vi "Power_Correlation9.vi"() -> ()   [LabVIEW 2021]
doc: "This VI opens a datalog file created with Write Datalog File Example.vi, reads one record at a time from the file until all are read, then closes the file and checks for errors. The record is a cluster containing a string and an array of single precision numbers."
uses:
  <vilib>/Analysis/2dsp.llb/Decimate (single shot, DBL).vi
  <vilib>/Analysis/baseanly.llb/Mean (DBL).vi
  Plot Routines.llb/Plot Globals.vi
  Response Analysis.llb/Analysis Globals.vi
  Display_Analysis.llb/Display & Avg Globals.vi
  Power_Correlation Utilities.llb/PowerCorrelation_globals.vi
  <vilib>/Analysis/NI_AALPro.lvlib
  <vilib>/Analysis/NI_AALBase.lvlib
panel:
  out "Trace B units":string
  out "Trace A units":string
  in  "Trace # 2":u8
  in  "Traces\nmV to uV":bool
  in  "redux factor":i32=30
  in  "sample rate redux of graph 2":bool
  out "Strings":T1
  out "Original Traces - all Chan":T2(array[cluster])
  out "Stat Results_Mean":T3
  in  "box filter graph":bool
  in  "single chan":bool=TRUE
  in  "Do Stats":bool
  in  "5 SD mark":bool
  out "Median Stats":T4
  out "Means":dbl[](array[numeric])
  in  "Pair":i32[](array[numeric])=[0, 1]
  in  "Export":bool
  in  "Value":enum16{"avg", "max", "min"}(ring)
  in  "Mode":enum16{"Indiv", "Mean SE"}(ring)
  in  "Analysis Transform":enum16{"None", "Log10"}(ring)
  out "Stat Plot":cluster{dbl[], dbl[]}[](graph)
  in  "Last #":i32=5
  in  "Shift by -500 except last traces":bool
  out "NewVal 2":variant
  out "Dual Parameters":T5 {"Depth B" format="%.2f"; "Depth A" format="%.2f"; "Cap B" format="%.2f"; "Cap A" format="%.2f"; "Comp B" format="%.2f"; "Comp A" format="%.2f"; "Extra Stim Mag B" format="%.2f"; "Extra Stim Mag A" format="%.2f"; "extra amp b" format="%.2f"; "extra amp a" format="%.2f"; "extra offset b" format="%.2f"; "extra offset a/cur" format="%.2f"; "extra dur" format="%.2f"; "extra mode" format="%.2f"; "Intra Stim Mag B" format="%.2f"; "Intra Stim Mag A" format="%.2f"; "Step Delay (sim)" format="%.2f"; "Step Amp B" format="%.2f"; "Rest Pot-B(mV)" format="%.2f"; "Rest Pot-A(mV)" format="%.2f"; "SR-B (MOhm)" format="%.2f"; "SR-A (MOhm)" format="%.2f"; "Clamp Level-B" format="%.2f"; "Clamp Level-A" format="%.2f"; "Gain-B" format="%.2f"; "Step/AI Offset(ms)" format="%.2f"; "Gain-A" format="%.2f"; "Post Stim Dur (ms)" format="%.2f"; "Test Interval(sec)" format="%.2f"; "Step Dur(ms)" format="%.2f"; "Step Amp" format="%.2f"; "Stim/AI Offset(ms)" format="%.2f"; "Pulse Number" format="%.2f"; "Pulse Interval(ms)" format="%.2f"; "Ext Stim Path" format="%.2f"; "Clamp Mode" format="%.2f"; "Current Rec Config" format="%.2f"; "Test Type" format="%.2f"}
  out "Analysis Notes":string
  in  "Trace Processing Params":T6={"X-Unit Factor"=enum."1", "dt change factor"=enum."1", "Box Filter Width"=5, "Filter"=enum."FIR lowpass", "Filter High Cut-off (Hz)"=0.2, "Filter Low Cut-off (Hz)"=300.0} {"Filter Low Cut-off (Hz)" format="%.2f"; "Filter High Cut-off (Hz)" format="%.2f"}
  in  "File Info":T7
  in  "Accumulate Func Plots":bool
  in  "Do Function":bool
  in  "Function":T8(ring)
  in  "cut mode":enum16{"Include", "Exclude"}(ring)
  out "dy B":sgl format="%.3f"
  out "dy A":sgl format="%.3f"
  out "File Paths":T9={"Data Path"=path "C:/", "Anal Path"=path "C:/", "File Path List"=[], "Listfile Path"=path "C:/", "Auto Anal Path"=path "C:/"}
  in  "Display Type":enum16{"Stim&Rec", "Dual", "Multi4", "Mapper"}(ring)=enum."Dual"
  in  "Trace B":T10(ring)=enum."File Tr 1"
  in  "Trace A":T10(ring)
  in  "Load Cursor Wind":bool
  in  "Dump Cursor Wind":bool
  in  "rectify":bool
  in  "Up State Analysis":bool
  in  "Export Name":string
  in  "Function post process":T11={"Freq range"={"min"=0.0, "max"=2000.0}, "Normalization"=enum."None", "Filter"={"Enabled"=FALSE, "Cutoff (cyc/Hz or Hz)"=0.4}} {"Filter"."Cutoff (cyc/Hz or Hz)" min=0 max=1000 step=0.0001 format="%.6f"; "Freq range"."max" format="%.2f"; "Freq range"."min" format="%.2f"}
  in  "Copy cursor window":bool
  in  "Func Mode":enum16{"Trace #", "Trace Ch"}(ring)=enum."Trace Ch"
  in  "Correlation Params":bool
  in  "Shuffle Trace":bool
  in  "cursor func":enum16{"2 filter", "+- 10%", "+- 5%", "+-2"}(ring)
  in  "cursors":bool
  in  "Func Type":enum16{"avg", "sum", "norm"}(ring)
  out "CV B":sgl=0.1 min=0 max=1 format="%.2f"
  out "CV A":sgl=0.1 min=0 max=1 format="%.2f"
  in  "Max Interval":sgl=1000.0 min=0 max=10000 format="%.2f"
  in  "Int Bin":sgl=1.0 min=0 max=100 format="%.2f"
  in  "AP Fract":sgl=0.1 min=0 max=1 format="%.2f"
  in  "AP Mode":enum16{"cor", "coh", "Int/AP"}(ring)
  in  "Zoom":bool
  in  "Cursor Near Spike":bool
  in  "Window":enum16{"all", "cursors"}(ring)
  in  "Spike Times B":T12(array[cluster]) {"t0" format="%.2f"; "Length (ms)" format="%.2f"; "Data" format="%.2f"}
  in  "Init Wind":bool
  in  "Spikes Times A":T12(array[cluster]) {"t0" format="%.2f"; "Length (ms)" format="%.2f"; "Data" format="%.2f"}
  in  "AP Time Course":bool
  in  "Add trace":bool
  in  "AP Freq Mode":enum16{"rates", "dif/avg", "all"}(ring)
  in  "AP Freq vs Time":bool
  in  "^2 four wind":bool
  out "Ran AP Cor":sgl format="%.3f"
  in  "Graph Mode":enum16{"Points", "Max", "Min"}(ring)=enum."Max"
  in  "Coord":enum16{"y", "z"}(ring)=enum."z"
  in  "Cursor Slave\nTime Course":bool
  in  "Graph Data":bool
  in  "Time Course Window":sgl=100.0 format="%.2f"
  in  "Function":T13(ring)
  in  "Init Data":bool
  out "y":sgl[](array[numeric]) format="%.2f"
  out "x":sgl[](array[numeric]) format="%.2f"
  out "Data":sgl[](array[numeric]) format="%.2f"
  in  "Add Datum":bool
  in  "Time Course Focus":enum16{"1", "2"}(ring)
  out "Time Course 2":sgl[][](graph)
  in  "Time Course Increment":i32=25
  in  "Time Course":bool
  out "Time Course 1":sgl[][](graph)
  in  "Spectrum Source":enum16{"Trace", "Function"}(ring)
  out "Function Units = ms?":bool
  in  "Filter":bool
  in  "Trace #":u8
  in  "Operate":bool
  in  "oper2":u8
  in  "oper1":u8
  in  "operation":T14(ring)=enum."mult"
  in  "Match dx read":bool
  out "dF":sgl=1.0 min=0 max=1000 step=0.1 format="%.3f"
  in  "Offset/Sc/Ph":sgl format="%.4f"
  in  "Component Num":i32
  in  "Function":T15(ring)
  out "Fixed Window Size":sgl=2000.0 format="%.2f"
  out "Window Size":sgl format="%.2f"
  in  "Fix Wind Size":bool
  in  "cut traces":bool
  in  "Normalization":enum16{"None", "Variance", "Sample Num"}(ring)=enum."Variance"
  in  "Assign Cursors In Plot":bool
  in  "One Cursor Window":bool=TRUE
  out "Cursor Windows by Trace":cluster{"start":dbl, "end":dbl}[](array[cluster]) {"end" format="%.1f"; "start" format="%.1f"}
  in  "Upper Factor":sgl=1.8 format="%.1f"
  in  "Lower Factor":sgl=1.4 format="%.1f"
  in  "Make window wrt Yel Cursor":bool
  out "Delta X":sgl format="%.2f"
  out "Graph 2 - cursor 0 x":sgl format="%.2f"
  out "Graph 2 - cursor 1 x":sgl format="%.2f"
  out "SD B":sgl format="%.5f"
  out "SD A":sgl format="%.5f"
  in  "scale":bool
  in  "Correllation Func":enum16{"labview", "Jay's"}(ring)=enum."Jay's"
  out "Window Avg":sgl format="%.8f"
  in  "Window Func":bool
  in  "Avg Pts":bool
  out "Delta Y":sgl format="%.3f"
  out "Pts Avg":sgl format="%.2f"
  in  "Get Red Cursonr Pts":bool
  in  "Pts Around Yellow cursor":sgl[](array[numeric]) format="%.1f"
  in  "Offset Traces":bool
  in  "Cutoff (cyc/Hz or Hz)":sgl=0.1 min=0 max=1000 step=0.0001 format="%.6f"
  out "Message":string
  in  "Filter Function":bool
  in  "Export Graph":T16(ring)
  in  "Fourier mode":bool
  in  "expand":bool
  in  "zoom":bool
  in  "Corr Func":enum16{"Auto", "Cross"}(ring)=enum."Cross"
  in  "Window Size (ms)":sgl=400.0 step=1 format="%.2f"
  in  "Set to B X-Axis":bool
  in  "Set to A X-Axis":bool
  in  "Prog Info":bool
  out "x-axis":string
  out "y-axis":string
  out "Window Constants":cluster{"Eq Noise BW":ext, "Coherent Gain":ext} {"Coherent Gain" format="%.2f"; "Eq Noise BW" format="%.2f"}
  in  "window":T17(ring)=enum."Hanning"
  out "samp/sec":sgl format="%.2f"
  in  "1/2 sample rate":bool
  in  "Std Function Parameters":T18={"Function"=2, "Mag/Phase"=0, "Magnitude Unit"=3, "Phase Unit"=0, " Log dB or Linear"=0} {"Log dB or Linear" items=["Linear", "dB", "dBm"]; "Phase Unit" items=["Degrees", "Radians"]; "Magnitude Unit" items=["Vrms", "Vpk", "Vrms^2", "Vpk^2", "Vrms/rtHz", "Vpk/rtHz", "Vrms^2/Hz", "Vpk^2/Hz"]; "Mag/Phase" items=["Magnitude", "Phase"]; "Function" items=["Time Waveform", "Amplitude Spectrum", "Power Spectrum", "Cross Power Spectrum", "Frequency Response", "Coherence", "Impulse Response"]}
  out "Focus Trace B":cluster{"T0":sgl, "Delta T":sgl, "Data":sgl[][]} {"Data" format="%.2f"; "Delta T" format="%.6f"; "T0" format="%.6f"}
  out "Focus Trace A":cluster{"T0":sgl, "Delta T":sgl, "Data":sgl[][]} {"Data" format="%.2f"; "Delta T" format="%.6f"; "T0" format="%.6f"}
  out "Old Focus":i32
  in  "Trace Ch Reference":enum16{"0", "1", "2", "3"}(ring)
  out "Trace B":T19(graph)={"T0"=0.0, "delta T"=0.19999999, "Individual Data Sweeps"=[]}
  in  "Focus":i32
  in  "Focus Mode":bool
  in  "Plot Flags 2":bool[](array[boolean])
  in  "Show All":bool
  in  "Trace Export":bool
  out "Graph 2":cluster{"T0":sgl, "delta T":sgl, sgl[][]}(graph)={"T0"=1.1399999, "delta T"=0.0001, []}
  in  "Load List File":bool
  in  "Get File List":bool
  in  "File Path List":cluster{"FilePath":path, "focus":bool}[](array[cluster])
  in  "Quit":bool
  out "Trace A":T19(graph)={"T0"=0.0, "delta T"=0.19999999, "Individual Data Sweeps"=[]}
  # "function\nInt Hist A\nInt Hist B"
  # "V=mV"
  # "Function Operations"
  # "Focus/Graph"
  # "MW, 1.282 = 0.2, 1.645 = 0.1, 1.960 = .05, 2.326 =.02, 2.576 = .01, 2.807 = .005, 3.090 = .002, 3.291 = .001"
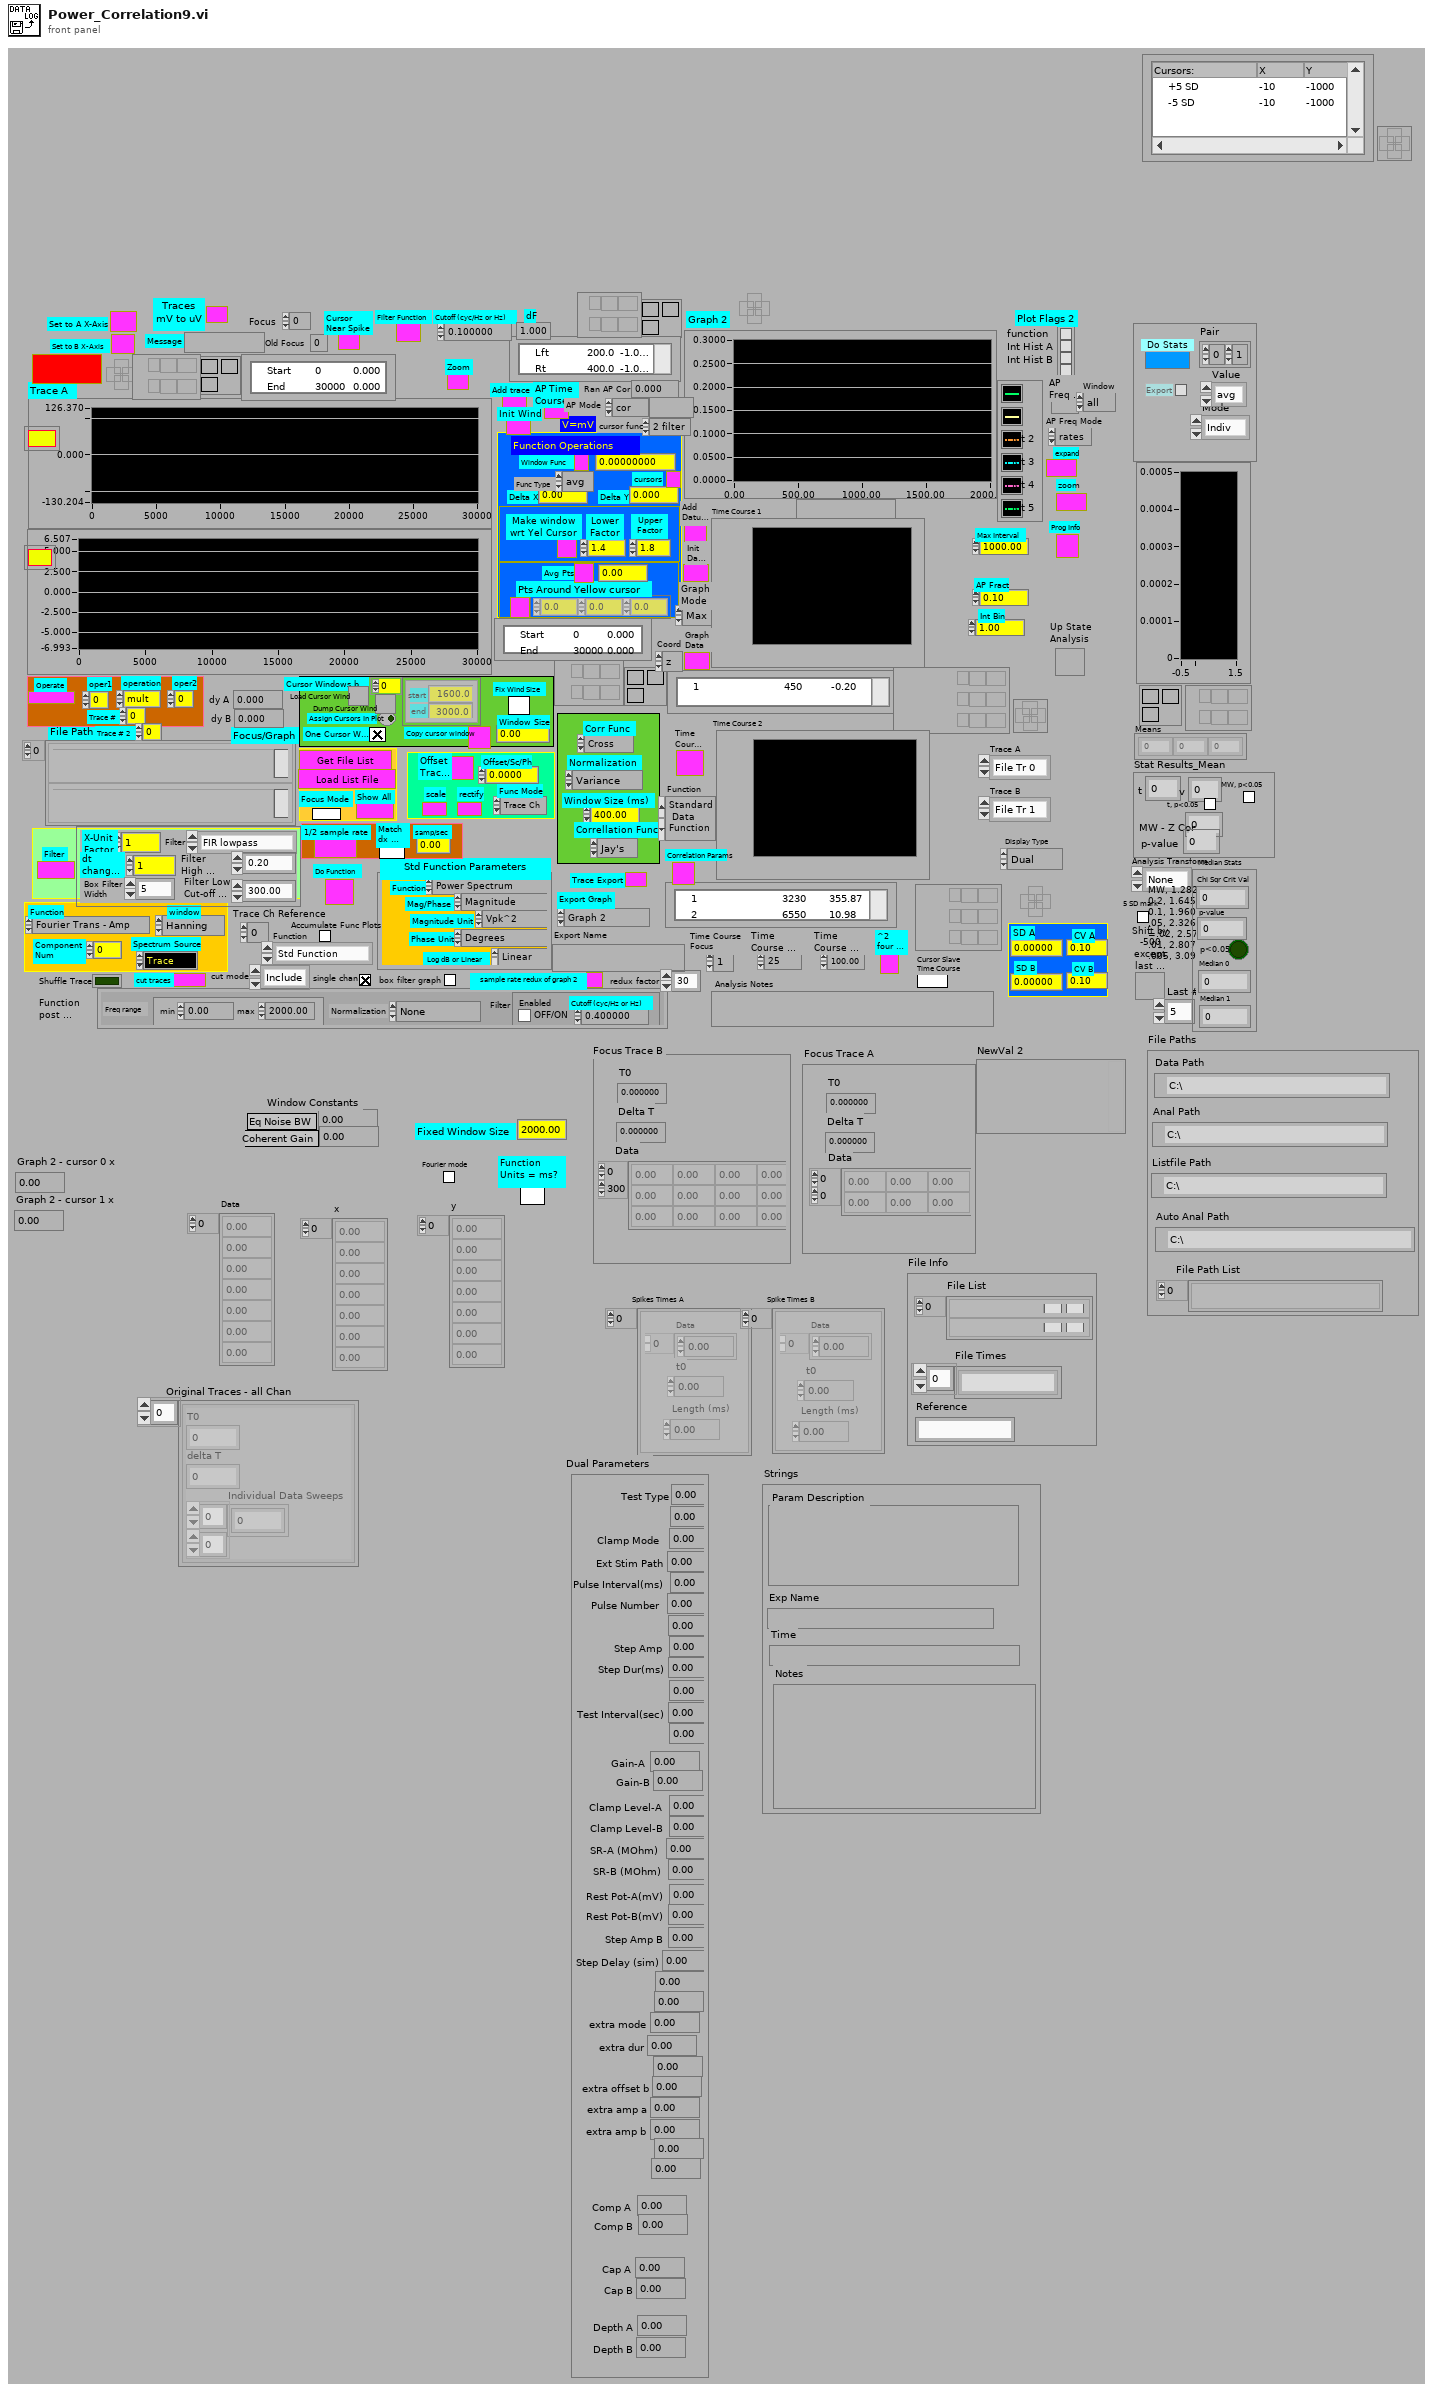
[diagram p1: front panel]
types:
  T1 = cluster{"Param Description":string, "Exp Name":string, "Time":string, "Notes":string}
  T2 = cluster{"T0":sgl, "delta T":sgl, "Individual Data Sweeps":sgl[][]}[]
  T3 = cluster{"t":dbl, "v":i32, "t, p<0.05":bool, "MW - Z Cor":dbl, "MW, p<0.05":bool, "p-value":dbl}
  T4 = cluster{"Chi Sqr Crit Val":dbl, "p-value":dbl, "p<0.05":bool, "Median 0":dbl, "Median 1":dbl}
  T5 = cluster{"Test Type":sgl, "Current Rec Config":sgl, "Clamp Mode":sgl, "Ext Stim Path":sgl, "Pulse Interval(ms)":sgl, "Pulse Number":sgl, "Stim/AI Offset(ms)":sgl, "Step Amp":sgl, "Step Dur(ms)":sgl, "Step/AI Offset(ms)":sgl, "Test Interval(sec)":sgl, "Post Stim Dur (ms)":sgl, "Gain-A":sgl, "Gain-B":sgl, "Clamp Level-A":sgl, "Clamp Level-B":sgl, "SR-A (MOhm)":sgl, "SR-B (MOhm)":sgl, "Rest Pot-A(mV)":sgl, "Rest Pot-B(mV)":sgl, "Step Amp B":sgl, "Step Delay (sim)":sgl, "Intra Stim Mag A":sgl, "Intra Stim Mag B":sgl, "extra mode":sgl, "extra dur":sgl, "extra offset a/cur":sgl, "extra offset b":sgl, "extra amp a":sgl, "extra amp b":sgl, "Extra Stim Mag A":sgl, "Extra Stim Mag B":sgl, "Comp A":sgl, "Comp B":sgl, "Cap A":sgl, "Cap B":sgl, "Depth A":sgl, "Depth B":sgl}
  T6 = cluster{"X-Unit Factor":enum16{"1000", "1"}, "dt change factor":enum16{"0.5", "1", "2", "4", "8", "16"}, "Box Filter Width":i16, "Filter":enum16{"None", "FIR lowpass", "FIR highpass", "FIR bandpass", "Box Avg", "Butterworth Bandpass", "Butterworth Highpass", "Butterworth Lowpass", "Butterworth Bandstop"}, "Filter High Cut-off (Hz)":dbl, "Filter Low Cut-off (Hz)":dbl}
  T7 = cluster{"File List":cluster{"File Name":string, "Display":bool, "Focus":bool}[], "File Times":string[], "Reference":string}
  T8 = enum16{"Std Function", "Correlation", "Correlation APs", "Fourier Trans", "Impulse Resp", "CV's", "SD's"}
  T9 = cluster{"Data Path":path, "Anal Path":path, "File Path List":path[], "Listfile Path":path, "Auto Anal Path":path}
  T10 = enum16{"File Tr 0", "File Tr 1", "File Tr 2", "File Tr 3"}
  T11 = cluster{"Freq range":cluster{"min":dbl, "max":dbl}, "Normalization":enum16{"sample norm", "area norm", "user limits", "None"}, "Filter":cluster{"Enabled":bool, "Cutoff (cyc/Hz or Hz)":sgl}}
  T12 = cluster{"Data":sgl[], "t0":sgl, "Length (ms)":sgl}[]
  T13 = enum16{"Standard Data Function", "Correlation", "AP Correlation", "Fourier Transform"}
  T14 = enum16{"add", "subtract", "mult", "div", "average"}
  T15 = enum16{"Fourier Trans - Amp", "Fourier Trans - Phase", "Reconstruct with FT"}
  T16 = enum16{"Graph 2", "traces (focus)", "All Traces (Ref)", "Color Graph 1"}
  T17 = enum16{"None ", "Hanning", "Hamming", "Blackman-Harris", "Exact Blackman", "Blackman", "Flat Top", "4 Term B-Harris ", "7 Term B-Harris"}
  T18 = cluster{"Function":u16, "Mag/Phase":u16, "Magnitude Unit":i32, "Phase Unit":u16, " Log dB or Linear":u16}
  T19 = cluster{"T0":sgl, "delta T":sgl, "Individual Data Sweeps":sgl[][]}
  T20 = cluster{"Task":enum16{"None", "Initialize", "Plot Traces", "Plot Graph2", "Read Data", "Variable Update", "Trace Plot Param"}, "Argument":i32}
  T21 = enum16{"None", "Initialize", "Plot Traces", "Plot Graph2", "Read Data", "Variable Update", "Trace Plot Param"}[]
  T22 = cluster{"File Path":path, "Start Path":path, "Prompt":string, "Pattern":string}
  T23 = enum16{"Interpolation", "Closest", "Closest (Windowed)"}
  T24 = enum32{"Lowpass", "Highpass", "Bandpass", "Bandstop"}
  T25 = enum16{"sample norm", "area norm", "user limits"}
  T26 = enum16{"Default - Within Graph Range", "Assign given coordinates"}
  T27 = enum16{"Within Graph Range", "X & Y coords", "Just X coords", "Just Y coords"}
  T28 = cluster{"+- factor*SD[0]":dbl, "+- factor*SD[1]":dbl}
  T29 = enum16{"open", "replace", "create", "open or create", "replace or create", "replace or create with confirmation"}
  T30 = enum16{"None", "Initialize", "Plot Traces", "Plot Graph2", "Read Data", "Variable Update", "Trace Plot Param"}
  T31 = cluster{"dt change factor":enum16{"0.5", "1", "2", "4", "8", "16"}, "X-Unit Factor":enum16{"1000", "1"}}
  T32 = cluster{"Exp Parameters":cluster{"Test Type":sgl, "Recording Config ":sgl, "Clamp Config":dbl[], "Ext Stim Path":sgl, "Pulse Interval(ms)":sgl, "Pulse Number":sgl, "Stim/AI Offset(ms)":sgl, "Step Amp":sgl, "Step Dur(ms)":sgl, "Step/AI Offset(ms)":sgl, "Test Interval(sec)":sgl, "Post Stim Dur (ms)":sgl, "Gain":sgl[], "Clamp Level":sgl[], "SR (MOhm)":sgl[], "Rest Pot {mV)":sgl[], "Step Amp B":sgl, "Step Delay (sim)":sgl, "Intra Stim Mag":sgl[], "extra mode":sgl, "extra dur":sgl, "extra offset a/cur":sgl, "extra offset b":sgl, "extra amp a":sgl, "extra amp b":sgl, "Extra Stim Mag A":sgl, "Extra Stim Mag B":sgl, "Comp A":sgl, "Comp B":sgl, "Cap A":sgl, "Cap B":sgl, "Depth A":sgl, "Depth B":sgl, "DAC Stim output":sgl}, "Strings":cluster{"Param Description":string, "Exp Name":string, "Time":string, "Notes":string}}
  T33 = cluster{"X0":sgl, "Delta X":sgl, "Data":sgl[][]}[]
  T34 = cluster{"Name":string, "Color":u32, "Style":u8, "Point Style":u8, "Name Visible":bool, "Allow Drag":bool, "Lock Style":u32, "Plot":u32, "Index":i32, "Position":cluster{"X":dbl, "Y":dbl}}[]
  T35 = typedef "LVCursorListTypeDef.ctl" = cluster{"Name":string, "Color":u32, "Style":u8, "Point Style":u8, "Name Visible":bool, "Allow Drag":bool, "Cursor Mode":u32, "Plot":i32, "Index":i32, "Position":cluster{"X":dbl, "Y":dbl}, "X Scale":u32, "Y Scale":u32, "Watch Plots":i32[], "Watch All Plots":bool, "Plot Area":i32, "Label Offset":cluster{"X":dbl, "Y":dbl}}[]
  T36 = cluster{"Corr Func":enum16{"Auto", "Cross"}, "Normalization":enum16{"None", "Variance", "Sample Num"}}
  T37 = cluster{"T0 (sec)":sgl, "dT (sec)":sgl, "Data":sgl[]}
  T38 = cluster{"Spike Threshold (mv)":sgl, "min interval flag":bool, "min interval (ms)":sgl, "Polarity":enum16{"Positive", "Negative"}}
  T39 = cluster{"Scaling":enum16{"Raw Count", "Norm by Ref Spike Count", "Norm by peak"}, "baseline Norm":enum16{"none", "subtract", "divide"}, "binsize":sgl, "Edge Correction":bool}
  T40 = cluster{i32, "Delta T":sgl, "Impulse Response":dbl[]}
  T41 = cluster{"Corr Func":enum16{"Auto", "Cross"}, "Window Size (ms)":sgl, "Normalization":enum16{"None", "Variance", "Sample Num"}}
  T42 = cluster{"Name":string, "Color":u32, "Hair Style":u8, "Point Style":u8, "Name Visible":bool, "Trackable":bool, "Lock Style":u32, "Plot Number":u32, "Marker Index":i32, "Location":cluster{"X":dbl, "Y":dbl}}[]
  T43 = typedef "LVOffsetAndMultiplierTypeDef.ctl" = cluster{"Offset":dbl, "Multiplier":dbl}
  T44 = cluster{"x":sgl, "XScale.Multiplier":dbl, dbl[][]}
  T45 = cluster{"Ref Wind Start (ms)":dbl, "Ref Wind End (ms)":dbl}
  T46 = cluster{"T0":sgl, "Delta T":sgl, "Data":sgl[][]}[]
  T47 = cluster{"Filter Low Cut-off (Hz)":dbl, sgl, "Filter High Cut-off (Hz)":dbl, sgl}
  T48 = cluster{string, u32, u8, u8, bool, bool, u32, u32, i32, cluster{dbl, dbl}}[]
  T49 = typedef "LVRangeTypeDef.ctl" = cluster{"Minimum":dbl, "Maximum":dbl, "Increment":dbl, "Minor Increment":dbl, "Start":dbl}
  T50 = typedef "LVMinMaxIncTypeDef.ctl" = cluster{"Minimum":dbl, "Maximum":dbl, "Increment":dbl}
  T51 = cluster{"Spike Times":sgl[], sgl, "Length (x-units)":sgl}
  T52 = cluster{"Spike Times":sgl[], "t0":sgl, "Length (x-units)":sgl}[]
  T53 = cluster{"T0 (sec)":sgl, "dT (sec)":sgl, "Data":sgl[]}[]
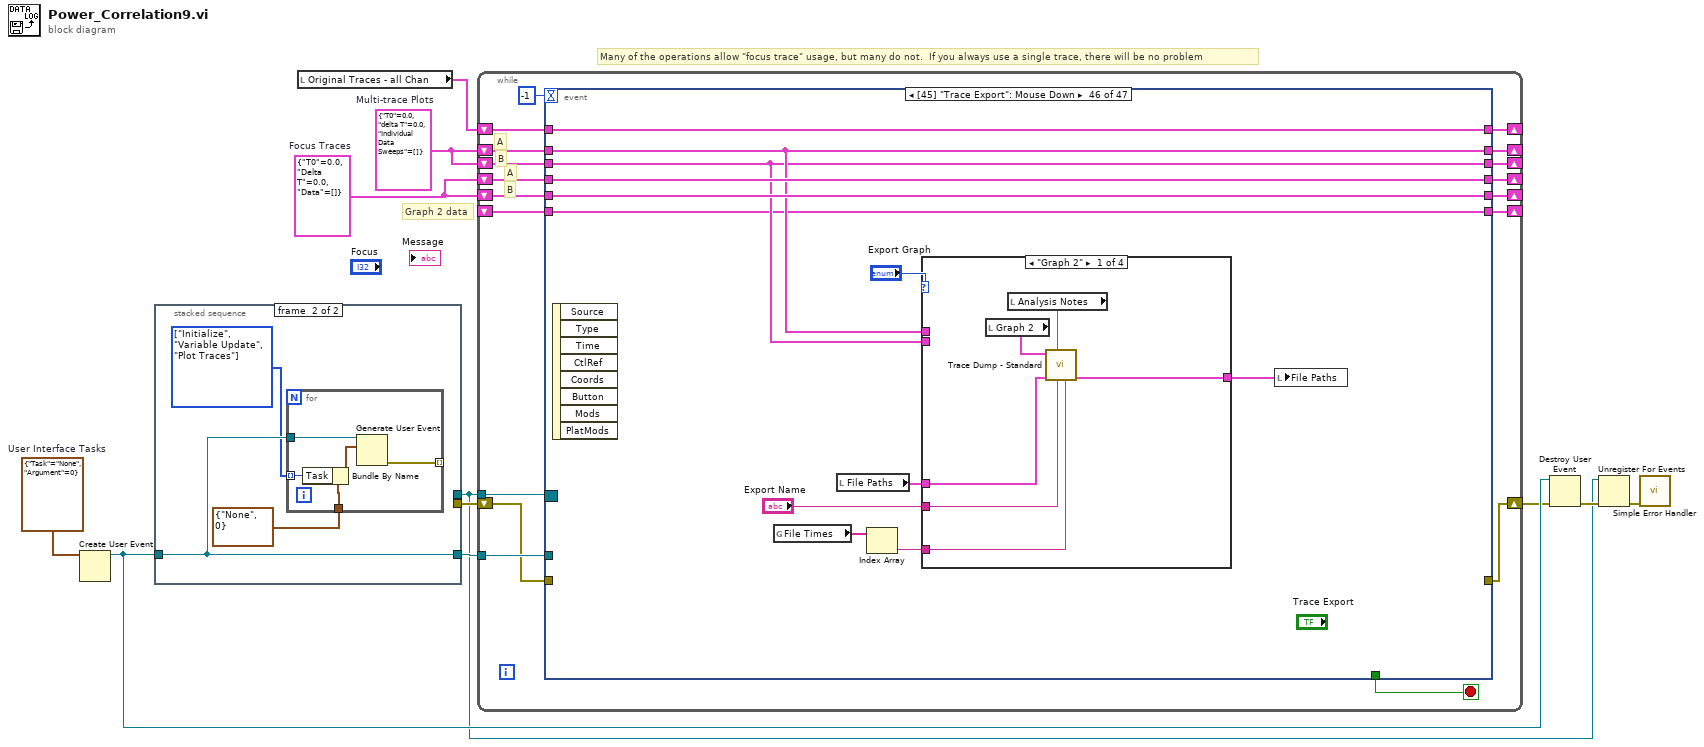
[diagram p0: block diagram]
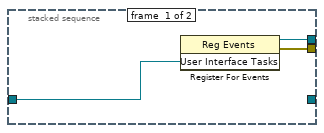
[diagram p2: hidden frame]
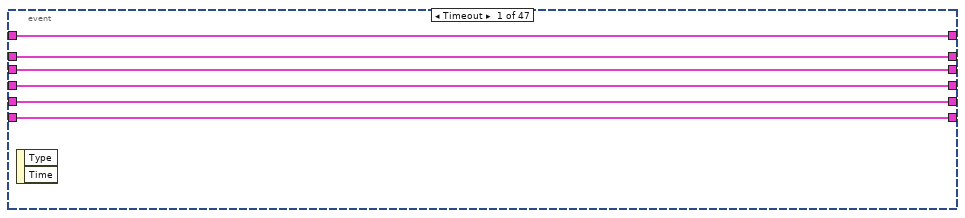
[diagram p3: hidden frame]
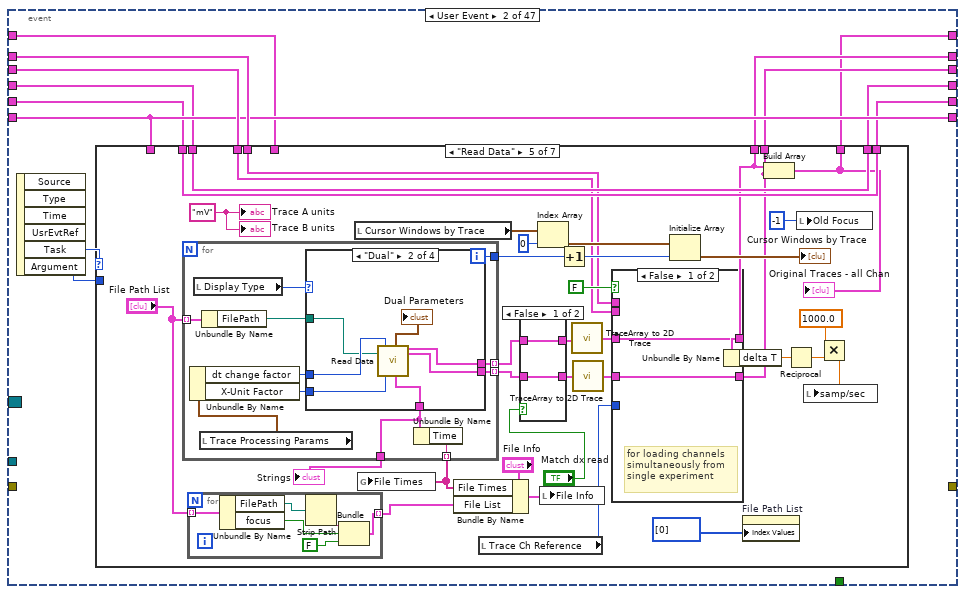
[diagram p4: hidden frame]
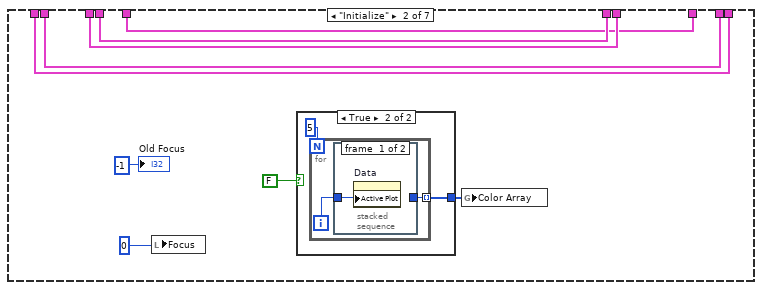
[diagram p6: hidden frame]
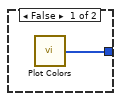
[diagram p7: hidden frame]
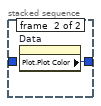
[diagram p8: hidden frame]
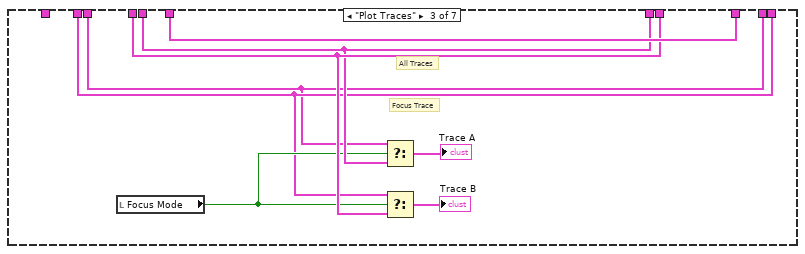
[diagram p9: hidden frame]
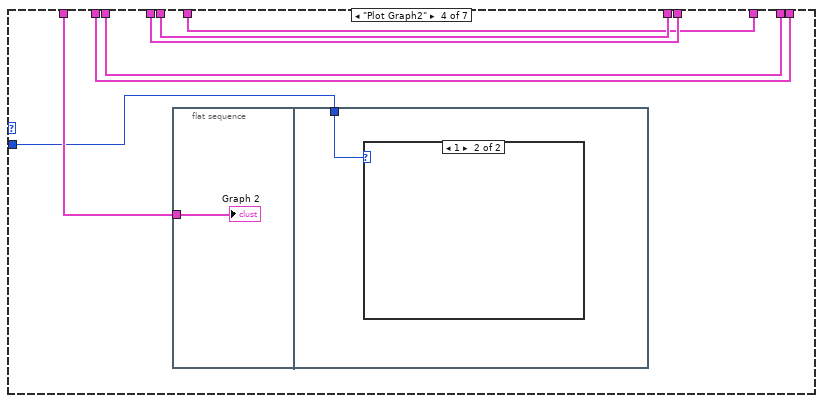
[diagram p10: hidden frame]
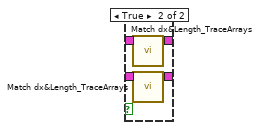
[diagram p14: hidden frame]
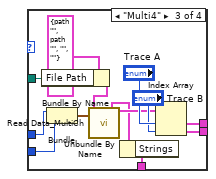
[diagram p16: hidden frame]
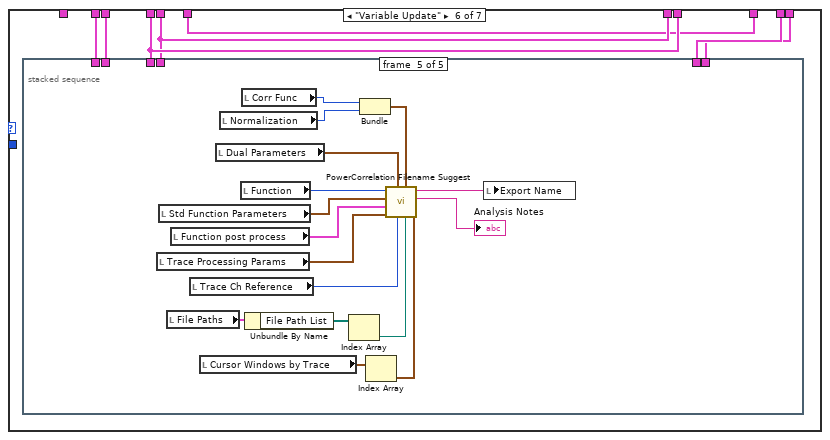
[diagram p18: hidden frame]
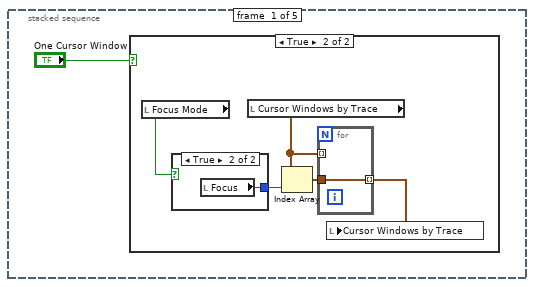
[diagram p19: hidden frame]
diagram:
  w9 = T20 {"Task"=enum."None", "Argument"=0}  # User Interface Tasks
  w10 = cluster{"T0":sgl, "Delta T":sgl, "Data":sgl[][]} {"T0"=0.0, "Delta T"=0.0, "Data"=[]}  # Focus Traces
  w11 = T19 {"T0"=0.0, "delta T"=0.0, "Individual Data Sweeps"=[]}  # Multi-trace Plots
  # "Graph 2 data"
  # "Many of the operations allow \"focus trace\" usage, but many do not.  If you always use a single trace, there will be no problem"
  n1 = Create User Event(user event datatype=w9) -> (user event=w4:refnum<user-event>)  [unwired: 1 in, 1 out]
  n2 = stacked-sequence {
    tunnel: [w14 _] -> w2
    tunnel: w4 -> [w13 w17]
    tunnel: [w12 _] -> w5
    tunnel: [_ w17] -> w8
    frame #0 {
      n3 = register-events(w13) -> (reference out=w14:refnum<event-registration>, error out=w12:errorcluster)  [unwired: 2 in]
    }
    frame #1 {
      w16 = T21 [enum."Initialize", enum."Variable Update", enum."Plot Traces"] items=["None", "Initialize", "Plot Traces", "Plot Graph2", "Read Data", "Variable Update", "Trace Plot Param"]
      n4 = for {
        tunnel: w17 -> [w22]
        tunnel: T20 {"Task"=enum."None", "Argument"=0} ("User Interface Tasks") -> [w20]
        tunnel: w16 -> [w19] mode=indexing
        tunnel: [w21] -> _ mode=indexing
        n5 = Bundle By Name(cluster=w20, "Task"=w19) -> (w18:T20)
        n6 = Generate User Event(user event=w22, event data cluster=w18) -> (error out=w21:errorcluster)  [unwired: 2 in, 1 out]
      }
    }
  }
  n7 = local read "Original Traces - all Chan"() -> (w1:T2)
  n8 = while {
    tunnel: w2 -> [w39]
    tunnel: w8 -> [w38]
    shift-right: [w34] -> _
    shift-left: w11 -> [w36]
    shift-right: [w33] -> _
    shift-left: w11 -> [w35]
    shift-right: [w30] -> _
    shift-left: w10 -> [w32]
    shift-right: [w29] -> _
    shift-left: w10 -> [w31]
    shift-right: [w25] -> w3
    shift-left: w5 -> [w26]
    shift-right: [w28] -> _
    shift-left: _ -> [w27]
    shift-right: [w23] -> _
    shift-left: w1 -> [w24]
    stop <- w40 stop-if-true
    # "B"
    # "B"
    # "A"
    # "A"
    n9 = event shown="[45] \"Trace Export\": Mouse Down" {
      selector: w39 -> [_ _ _ _ _ _ _ _ _ _ _ _ _ _ _ _ _ _ _ _ _ _ _ _ _ _ _ _ _ _ _ _ _ _ _ _ _ _ _ _ _ _ _ _ _ _ _]
      dyn-events: _ -> [_ _ _ _ _ _ _ _ _ _ _ _ _ _ _ _ _ _ _ _ _ _ _ _ _ _ _ _ _ _ _ _ _ _ _ _ _ _ _ _ _ _ _ _ _ _ _]
      timeout: -1 -> [_ _ _ _ _ _ _ _ _ _ _ _ _ _ _ _ _ _ _ _ _ _ _ _ _ _ _ _ _ _ _ _ _ _ _ _ _ _ _ _ _ _ _ _ _ _ _]
      tunnel: [_ _ _ _ _ _ _ _ _ _ _ _ _ _ _ _ _ _ _ _ _ _ _ _ _ _ _ _ _ _ _ _ _ _ _ _ _ _ _ _ _ _ _ _ _ _ w1683] -> w40
      tunnel: w38 -> [_ _ w313 w341 w363 w396 _ w422 w442 w484 w698 _ _ _ w840 w905 w951 _ w1005 w1031 w1059 _ _ w1117 _ _ w1195 w1253 _ w1278 w1316 _ _ _ w1392 _ _ _ _ _ _ w1578 _ _ _ _ _]
      tunnel: w36 -> [w46 w58 w318 w348 w367 w393 w413 w428 w458 w492 w704 w711 w753 w826 w844 w909 w964 w1003 w1023 w1041 w1063 w1077 w1091 w1125 w1162 w1181 w1200 w1231 w1273 w1285 w1320 w1350 w1377 w1390 w1402 w1426 w1462 w1469 w1502 _ w1548 w1584 w1591 w1602 w1614 w1622 w1682]
      tunnel: w35 -> [w45 w57 w317 w347 w366 w392 w412 w427 w457 w491 w703 w710 w752 w825 w843 w908 w963 w1002 w1022 w1040 w1062 w1076 w1090 w1124 w1161 w1180 w1199 w1230 w1272 w1284 w1319 w1349 w1376 w1389 w1401 w1425 w1461 w1468 w1503 w1536 w1547 w1583 w1590 w1601 w1613 w1621 w1681]
      tunnel: [w46 w50 w318 w348 w365 w393 w413 w428 w458 w492 w704 w711 w753 w826 w842 w907 w962 w1003 w1023 w1039 w1061 w1077 w1091 w1125 w1162 w1181 w1198 w1232 w1273 w1285 w1320 w1350 w1377 w1390 w1400 w1426 w1462 w1469 w1502 w1534 w1548 w1584 w1591 w1602 w1614 w1622 w1682] -> w34
      tunnel: [w45 w49 w317 w347 w364 w392 w412 w427 w457 w491 w703 w710 w752 w825 w841 w906 w961 w1002 w1022 w1038 w1060 w1076 w1090 w1124 w1161 w1180 w1197 w1229 w1272 w1284 w1319 w1349 w1376 w1389 w1399 w1425 w1461 w1468 w1503 w1536 w1547 w1583 w1590 w1601 w1613 w1621 w1681] -> w33
      tunnel: w32 -> [w44 w53 w316 w346 w378 w399 w411 w425 w446 w490 w702 w708 w751 w824 w847 w911 w967 w1001 w1021 w1047 w1069 w1075 w1089 w1123 w1160 w1179 w1196 w1254 w1271 w1283 w1318 w1348 w1375 w1380 w1415 w1424 w1460 w1467 w1501 w1535 w1546 w1582 w1589 w1604 w1612 w1626 w1680]
      tunnel: w31 -> [w43 w54 w315 w345 w377 w398 w410 w424 w445 w489 w701 w707 w750 w823 w846 w910 w966 w1000 w1020 w1046 w1068 w1074 w1088 w1122 w1159 w1178 w1201 w1255 w1270 w1282 w1317 w1347 w1374 w1388 w1414 w1423 w1459 w1466 w1500 w1533 w1545 w1581 w1588 w1605 w1611 w1625 w1679]
      tunnel: [w44 w52 w316 w346 w378 w399 w411 w425 w446 w490 w702 w708 w751 w824 w847 w911 w967 w1001 w1021 w1047 w1069 w1075 w1089 w1123 w1160 w1179 w1196 w1254 w1271 w1283 w1318 w1348 w1375 w1380 w1415 w1424 w1460 w1467 w1501 w1534 w1546 w1582 w1589 w1604 w1612 w1626 w1680] -> w30
      tunnel: [w43 w51 w315 w345 w377 w398 w410 w424 w445 w489 w701 w707 w750 w823 w846 w910 w966 w1000 w1020 w1046 w1068 w1074 w1088 w1122 w1159 w1178 w1201 w1255 w1270 w1282 w1317 w1347 w1374 w1388 w1414 w1423 w1459 w1466 w1500 w1533 w1545 w1581 w1588 w1605 w1611 w1625 w1679] -> w29
      tunnel: [w42 w56 w309 w338 w360 w390 w405 w426 w444 w487 w700 w706 w746 w817 w837 w903 w960 w999 w1007 w1037 w1057 w1071 w1079 w1119 w1158 w1176 w1193 w1251 w1267 w1280 w1314 w1346 w1370 w1379 w1394 w1419 w1458 w1465 w1499 w1532 w1542 w1580 w1586 w1606 w1608 w1620 w1678] -> w28
      tunnel: w27 -> [w42 w56 w309 w338 w360 w391 w405 w426 _ w486 w700 w706 w746 w817 w837 w903 w960 w999 _ w1037 w1057 w1071 w1079 w1120 w1158 w1176 w1193 w1251 w1267 w1280 w1314 w1346 w1370 w1379 _ w1419 w1458 w1465 w1499 w1532 w1542 w1580 w1586 w1606 w1608 w1620 w1678]
      tunnel: w26 -> [_ _ w308 _ _ _ _ w421 _ _ _ _ _ _ _ _ w950 _ _ w1035 _ _ _ _ _ _ _ w1237 _ _ _ _ _ _ _ _ _ _ _ _ _ _ _ _ _ _ _]
      tunnel: [_ _ w307 _ _ _ _ w420 _ _ _ _ _ _ _ _ w949 _ _ w1034 _ _ _ _ _ _ _ w1236 _ _ _ _ _ _ _ _ _ _ _ _ _ _ _ _ _ _ _] -> w25
      tunnel: w24 -> [w41 w47 w306 w337 w359 w394 w404 w418 w441 w468 w697 w705 w745 w816 w836 w902 w948 w998 w1004 w1030 w1056 w1070 w1078 w1114 w1157 w1175 w1192 w1228 w1266 w1277 w1313 w1322 w1369 w1378 w1391 w1418 w1457 w1464 w1498 w1531 w1540 w1577 w1585 w1599 w1607 w1615 w1677]
      tunnel: [w41 w48 w306 w337 w359 w394 w404 w418 w441 w468 w697 w705 w745 w816 w836 w902 w948 w998 w1004 w1030 w1056 w1070 w1078 w1114 w1157 w1175 w1192 w1228 w1266 w1277 w1313 w1322 w1369 w1378 w1391 w1418 w1457 w1464 w1498 w1531 w1540 w1577 w1585 w1599 w1607 w1615 w1677] -> w23
      event Timeout {
        n10 = event-data() -> ()  [unwired: 3 out]
      }
      event User Event {
        n11 = event-data() -> ("Task"=w59:T30, "Argument"=w55:i32)  [unwired: 5 out]
        n12 = case shown="\"Read Data\"" w59 {
          tunnel: [w64 w73 w84 w95 w102 w193 w295] -> w50
          tunnel: [w63 w72 w85 w94 w101 w194 w294] -> w49
          tunnel: w58 -> [w64 w73 w84 w95 w104 w193 w295]
          tunnel: w57 -> [w63 w72 w85 w94 w103 w194 w294]
          tunnel: w56 -> [_ _ _ w93 _ _ _]
          tunnel: w55 -> [_ _ _ w92 _ _ _]
          tunnel: w54 -> [w62 w68 w82 w91 w115 w191 w292]
          tunnel: w53 -> [w61 w67 w81 w90 w114 w192 w293]
          tunnel: [w61 w67 w81 w90 w114 w190 w293] -> w52
          tunnel: [w62 w68 w82 w91 w115 w189 w292] -> w51
          tunnel: [w60 w65 w86 w89 w100 w188 w291] -> w48
          tunnel: w47 -> [w60 w65 w86 w89 _ w188 w291]
          frame "None", Default {
          }
          frame "Initialize" {
            n13 = local write "Focus"(0 ("Focus")) -> ()
            n14 = case shown="True" FALSE {
              tunnel: [w74 w75] -> w70
              frame False {
                n15 = call "Plot Colors.vi"() -> ("Color Array"=w74:u32[])
              }
              frame True {
                n16 = for {
                  N: 5 -> [_]
                  tunnel: [w77] -> w75 mode=indexing
                  i -> [w78]
                  n17 = stacked-sequence {
                    tunnel: w78 -> [w79 _]
                    tunnel: [_ w80] -> w77
                    frame #0 {
                      n18 = property on="Data" class="WFGraph (strict)"("Active Plot"=w79) -> ()  [unwired: 2 in, 2 out]
                    }
                    frame #1 {
                      n19 = property on="Data" class="WFGraph (strict)"() -> ("Plot.Plot Color"=w80:u32)  [unwired: 2 in, 2 out]
                    }
                  }
                }
              }
            }
            n20 = global write "Plot Globals.vi" "Color Array"(w70) -> ()
            "Old Focus" <- -1 ("Old Focus")
          }
          frame "Plot Traces" {
            # "All Traces"
            # "Focus Trace"
            n21 = local read "Focus Mode"() -> (w83:bool)
            n22 = Select(t=w81, s=w83, f=w84) -> (s? t:f=→"Trace A":T19)
            n23 = Select(t=w82, s=w83, f=w85) -> (s? t:f=→"Trace B":T19)
          }
          frame "Plot Graph2" {
            n24 = flat-sequence {
              tunnel: w93 -> [w96]
              tunnel: w92 -> [w97]
              frame #0 {
                "Graph 2" <- w96
              }
              frame #1 {
                n25 = case shown="1" w97 {
                  frame 0, Default {
                  }
                  frame 1 {
                  }
                }
              }
            }
          }
          frame "Read Data" {
            w98 = "mV" ("Trace A units")
            n26 = for {
              tunnel: "File Path List" -> [w167] mode=indexing
              tunnel: [w166] -> w132
              tunnel: [w163] -> w127 mode=indexing
              tunnel: [w162] -> w126 mode=indexing
              tunnel: [w165] -> w110 mode=indexing
              tunnel: [w157] -> w99
              i -> [w166]
              n27 = local read "Display Type"() -> (w161:enum16{"Stim&Rec", "Dual", "Multi4", "Mapper"})
              n28 = local read "Trace Processing Params"() -> (w160:T6)
              n29 = Unbundle By Name(w160) -> ("dt change factor"=w158:enum16{"0.5", "1", "2", "4", "8", "16"}, "X-Unit Factor"=w159:enum16{"1000", "1"})
              n30 = Unbundle By Name(w167) -> ("FilePath"=w164:path)
              n31 = case shown="\"Dual\"" w161 {
                tunnel: w164 -> [_ w173 w178 _]
                tunnel: w159 -> [_ w172 w181 _]
                tunnel: w158 -> [_ w174 w182 _]
                tunnel: [_ w169 w175 _] -> w157
                tunnel: [_ w171 w184 _] -> w163
                tunnel: [_ w170 w183 _] -> w162
                frame "Stim&Rec", Default {
                }
                frame "Dual" {
                  n32 = call "Read Data.vi"("File Path In"=w173, "dt change factor"=w174, "X-Unit Factor"=w172) -> ("Dual Parameters"=→"Dual Parameters":T5, "Strings"=w169:T1, "Trace 1"=w171:cluster{"T0":sgl, "dT":sgl, "Data":sgl[]}, "Trace 2"=w170:cluster{"T0":sgl, "dT":sgl, "Data":sgl[]})  [unwired: 5 in, 8 out]
                }
                frame "Multi4" {
                  n33 = Bundle By Name(cluster=T22 {"File Path"=path "", "Start Path"=path "", "Prompt"="", "Pattern"=""} ("File Path Info In"), "File Path"=w178) -> (w177:T22)
                  n34 = Bundle("dt change factor"=w182, "X-Unit Factor"=w181) -> (w180:T31)  [unwired: 1 in]
                  n35 = call "Read Data_MultiCh.vi"("File Path Info In"=w177, "Trace Modifications"=w180) -> ("Exp Info"=w176:T32, "Trace Array"=w185:cluster{"T0":sgl, "dT":sgl, "Data":sgl[]}[])  [unwired: 4 in, 12 out]
                  n36 = Unbundle By Name(w176) -> ("Strings"=w175:T1)
                  n37 = Index Array(array=w185, index #1="Trace A", index #2="Trace B") -> (element #1=w184:cluster{"T0":sgl, "dT":sgl, "Data":sgl[]}, element #2=w183:cluster{"T0":sgl, "dT":sgl, "Data":sgl[]})
                }
                frame "Mapper" {
                }
              }
              n38 = Unbundle By Name(w157) -> ("Time"=w165:string)
            }
            "Strings" <- w99
            n39 = for {
              tunnel: "File Path List" -> [w150] mode=indexing
              tunnel: [w148] -> w111 mode=indexing
              n40 = Unbundle By Name(w150) -> ("FilePath"=w146:path, "focus"=w149:bool)
              n41 = Strip Path(path=w146) -> (name=w145:string)  [unwired: 1 out]
              n42 = Bundle("name"=w145, "focus"=w149, FALSE) -> (w148:cluster{"name":string, "focus":bool, bool})  [unwired: 1 in]
            }
            n43 = local read "Cursor Windows by Trace"() -> (w129:cluster{"start":dbl, "end":dbl}[])
            n44 = global write "Analysis Globals.vi" "File Times"(w110) -> ()
            n45 = Bundle By Name(cluster="File Info", "File Times"=w110, "File List"=w111) -> (w109:T7)
            n46 = local read "Trace Ch Reference"() -> (w105:enum16{"0", "1", "2", "3"})
            n47 = case shown="False" "Match dx read" {
              tunnel: w126 -> [w151 w156]
              tunnel: w127 -> [w152 w155]
              tunnel: [w152 w154] -> w124
              tunnel: [w151 w153] -> w123
              frame False {
              }
              frame True {
                n48 = call <userlib>:"Match dx&Length_TraceArrays.vi"("Trace Array In"=w155) -> ("Trace Array Out"=w154:cluster{"X0":sgl, "Delta X":sgl, "Data":sgl[]}[])  [unwired: 3 in, 1 out]
                n49 = call <userlib>:"Match dx&Length_TraceArrays.vi"("Trace Array In"=w156) -> ("Trace Array Out"=w153:cluster{"X0":sgl, "Delta X":sgl, "Data":sgl[]}[])  [unwired: 3 in, 1 out]
              }
            }
            n50 = Index Array(array=w129, index=0) -> (element=w128:cluster{"start":dbl, "end":dbl})
            n51 = local write "File Info"(w109) -> ()
            n52 = Increment(x=w132) -> (x+1=w131:i32)
            n53 = call <userlib>:"TraceArray to 2D Trace.vi"("Trace Array"=w124) -> ("2D Trace"=w106:cluster{"X0":sgl, "Delta X":sgl, "Data":sgl[][]})
            n54 = call <userlib>:"TraceArray to 2D Trace.vi"("Trace Array"=w123) -> ("2D Trace"=w107:cluster{"X0":sgl, "Delta X":sgl, "Data":sgl[][]})
            n55 = case shown="False" FALSE {
              tunnel: w107 -> [w134 _]
              tunnel: w106 -> [w133 w139]
              tunnel: [w134 w135] -> w101
              tunnel: [w133 w138] -> w102
              tunnel: w105 -> [_ w140]
              tunnel: w104 -> [_ w137]
              tunnel: w103 -> [_ w136]
              frame False {
                # "for loading channels\nsimultaneously from\nsingle experiment"
              }
              frame True {
                # "for loading each chan\nindividually from different exp's"
                n56 = case shown="\"0\", Default" w140 {
                  tunnel: w139 -> [w142 w144]
                  tunnel: [w142 w143] -> w138
                  tunnel: w137 -> [_ w143]
                  tunnel: w136 -> [w141 _]
                  tunnel: [w141 w144] -> w135
                  frame "0", Default {
                  }
                  frame "1" {
                  }
                }
              }
            }
            n57 = Initialize Array "Initialize Array"(w128, w131) -> (→"Cursor Windows by Trace":cluster{"start":dbl, "end":dbl}[])
            n58 = Unbundle By Name(w102) -> ("delta T"=w122:sgl)
            n59 = property on="File Path List" class="Arr (strict)"("Index Values"=u32[] [0]) -> ()  [unwired: 2 in, 2 out]
            n60 = Build Array(w102, w101) -> (w100:T33)
            "Original Traces - all Chan" <- w100
            n61 = Reciprocal(x=w122) -> (1/x=w121:sgl)
            n62 = local write "Old Focus"(-1 ("Old Focus")) -> ()
            n63 = Multiply(x=sgl 1000.0, y=w121) -> (x*y=w120:sgl)
            n64 = local write "samp/sec"(w120) -> ()
            "Trace A units" <- w98
            "Trace B units" <- w98
          }
          frame "Variable Update" {
            n65 = stacked-sequence {
              tunnel: w194 -> [_ _ w233 _ _]
              tunnel: w193 -> [_ _ w232 _ _]
              tunnel: w192 -> [_ _ w231 _ _]
              tunnel: w191 -> [_ _ w230 _ _]
              tunnel: [_ _ w229 _ _] -> w190
              tunnel: [_ _ w228 _ _] -> w189
              frame #0 {
                n66 = case shown="True" "One Cursor Window" {
                  frame False {
                  }
                  frame True {
                    n67 = local read "Focus Mode"() -> (w197:bool)
                    n68 = case shown="True" w197 {
                      tunnel: [0 w202] -> w196
                      frame False {
                      }
                      frame True {
                        n69 = local read "Focus"() -> (w202:i32)
                      }
                    }
                    n70 = local read "Cursor Windows by Trace"() -> (w200:cluster{"start":dbl, "end":dbl}[])
                    n71 = Index Array(array=w200, index=w196) -> (element=w199:cluster{"start":dbl, "end":dbl})
                    n72 = for {
                      tunnel: w200 -> [_] mode=indexing
                      tunnel: w199 -> [w203]
                      tunnel: [w203] -> w198 mode=indexing
                    }
                    n73 = local write "Cursor Windows by Trace"(w198) -> ()
                  }
                }
              }
              frame #1 {
                n74 = local read "File Path List"() -> (w213:cluster{"FilePath":path, "focus":bool}[])
                n75 = property on="Graph 2" class="WFGraph (strict)"() -> ("Old Cursor List"=w212:T34)  [unwired: 2 in, 2 out]
                n76 = for {
                  tunnel: w213 -> [w227] mode=indexing
                  tunnel: [w226] -> w214 mode=indexing
                  n77 = Unbundle By Name(w227) -> ("focus"=w226:bool)
                }
                n78 = call "graphCursor_info.vi"("Cursor List"=w212) -> ("dy"=→"Delta Y":sgl, "dx"=→"Delta X":sgl, "x1"=→"Graph 2 - cursor 1 x":dbl, "x0"=→"Graph 2 - cursor 0 x":dbl)  [unwired: 1 in, 6 out]
                n79 = global write "Plot Globals.vi" "Resp Plots 1"(w214) -> ()
                n80 = local read "Fixed Window Size"() -> (w205:sgl)
                n81 = Less Than 0?(x=w205) -> (x < 0?=w204:bool)
                n82 = And(x="Fix Wind Size", y=w204) -> (x .and. y?=w206:bool)
                n83 = case shown="False" w206 {
                  tunnel: "Fix Wind Size" -> [w215 _]
                  frame False {
                    n84 = case shown="False" w215 {
                      frame False {
                        n85 = local write "Fixed Window Size"(sgl -1.0 ("Fixed Window Size")) -> ()
                      }
                      frame True {
                      }
                    }
                  }
                  frame True {
                    n86 = local read "Cursor Windows by Trace"() -> (w222:cluster{"start":dbl, "end":dbl}[])
                    n87 = local read "Focus Mode"() -> (w223:bool)
                    n88 = case shown="False" w223 {
                      tunnel: [0 ("Focus") w225] -> w221
                      frame False {
                      }
                      frame True {
                        n89 = local read "Focus"() -> (w225:i32)
                      }
                    }
                    n90 = Index Array(array=w222, index=w221) -> (element=w220:cluster{"start":dbl, "end":dbl})
                    n91 = Unbundle By Name(w220) -> ("end"=w219:dbl, "start"=w218:dbl)
                    n92 = Subtract(x=w219, y=w218) -> (x-y=→"Fixed Window Size":dbl)
                  }
                }
              }
              frame #2 {
                n93 = case shown="False" "Focus Mode" {
                  tunnel: w233 -> [_ w256]
                  tunnel: w232 -> [_ w255]
                  tunnel: w231 -> [w236 w247]
                  tunnel: w230 -> [w235 _]
                  tunnel: [w236 w249] -> w229
                  tunnel: [w235 w248] -> w228
                  frame False {
                    n94 = local read "Old Focus"() -> (w237:i32)
                    n95 = Greater Or Equal To 0?(x=w237) -> (x >= 0?=w238:bool)
                    n96 = case shown="True" w238 {
                      frame False {
                      }
                      frame True {
                        n97 = local write "Assign Cursors In Plot"(TRUE ("Assign Cursors Flag")) -> ()
                        n98 = local write "Old Focus"(-1 ("Old Focus")) -> ()
                      }
                    }
                  }
                  frame True {
                    w251 = 1 ("length")
                    n99 = global read "Plot Globals.vi" "Resp Plots 1"() -> (w258:bool[])
                    n100 = local read "Focus"() -> (w257:i32)
                    n101 = Unbundle By Name(w255) -> ("T0"=w246:sgl, "delta T"=w245:sgl, "Individual Data Sweeps"=w254:sgl[][])
                    n102 = call "Update Focus Flags.vi"("Current Focus"=w257, "Focus Flags"=w258) -> ("New Focus"=w241:i32, "New Focus Flags"=w261:bool[])  [unwired: 3 in, 3 out]
                    n103 = Unbundle By Name(w256) -> ("Individual Data Sweeps"=w252:sgl[][])
                    n104 = Increment(x=w241) -> (x+1=w243:i32)
                    n105 = Build Array(w241, w243) -> (w242:i32[])
                    n106 = local write "Focus"(w241) -> ()
                    n107 = property on="Cursor Windows by Trace" class="Arr (strict)"("Index Values"=w242) -> ()  [unwired: 2 in, 2 out]
                    n108 = local read "File Path List"() -> (w260:cluster{"FilePath":path, "focus":bool}[])
                    n109 = Bundle By Name(cluster=w247, "T0"=w246, "Delta T"=w245) -> (w244:cluster{"T0":sgl, "Delta T":sgl, "Data":sgl[][]})
                    n110 = Delete From Array "Delete From Array"(array=w254, length=w251, index (row)=w241) -> (deleted portion=w253:sgl[][])  [unwired: 1 in, 1 out]
                    n111 = Delete From Array(array=w252, length=w251, index (row)=w241) -> (deleted portion=w250:sgl[][])  [unwired: 1 in, 1 out]
                    n112 = for {
                      tunnel: w261 -> [w263] mode=indexing
                      tunnel: w260 -> [w264] mode=indexing
                      tunnel: [w262] -> w259 mode=indexing
                      n113 = Bundle By Name(cluster=w264, "focus"=w263) -> (w262:cluster{"FilePath":path, "focus":bool})
                    }
                    n114 = Bundle By Name(cluster=w244, "Data"=w250) -> (w248:cluster{"T0":sgl, "Delta T":sgl, "Data":sgl[][]})
                    n115 = Bundle By Name(cluster=w244, "Data"=w253) -> (w249:cluster{"T0":sgl, "Delta T":sgl, "Data":sgl[][]})
                    n116 = global write "Plot Globals.vi" "Resp Plots 1"(w261) -> ()
                    n117 = local write "File Path List"(w259) -> ()
                  }
                }
                "Focus Trace A" <- w229
                "Focus Trace B" <- w228
              }
              frame #3 {
                n118 = case shown="True" "Assign Cursors In Plot" {
                  frame False {
                  }
                  frame True {
                    n119 = property on="Cursor Windows by Trace" class="Arr (strict)"() -> ("Index Values"=w272:u32[])  [unwired: 2 in, 2 out]
                    n120 = local read "Cursor Windows by Trace"() -> (w274:cluster{"start":dbl, "end":dbl}[])
                    n121 = Index Array(array=w272, index=0 ("Index")) -> (element=w271:u32)
                    n122 = Index Array(array=w274, index=w271) -> (element=w270:cluster{"start":dbl, "end":dbl})
                    n123 = property on="Trace B" class="WFGraph (strict)"() -> ("CrsrList"=w266:T35)  [unwired: 2 in, 2 out]
                    n124 = property on="Trace A" class="WFGraph (strict)"() -> ("CrsrList"=w267:T35)  [unwired: 2 in, 2 out]
                    n125 = call "Assign Cursor Coordinates_LV8.vi"("X Coords"=w270, "Cursor List In"=w266) -> ("Cursor List Out"=w268:T35)  [unwired: 7 in, 2 out]
                    n126 = call "Assign Cursor Coordinates_LV8.vi"("X Coords"=w270, "Cursor List In"=w267) -> ("Cursor List Out"=w269:T35)  [unwired: 7 in, 2 out]
                    n127 = property on="Trace A" class="WFGraph (strict)"("CrsrList"=w269) -> ()  [unwired: 2 in, 2 out]
                    n128 = property on="Trace B" class="WFGraph (strict)"("CrsrList"=w268) -> ()  [unwired: 2 in, 2 out]
                  }
                }
              }
              frame #4 {
                n129 = local read "Trace Processing Params"() -> (w284:T6)
                n130 = local read "Std Function Parameters"() -> (w288:T18)
                n131 = local read "File Paths"() -> (w279:T9)
                n132 = local read "Function post process"() -> (w287:T11)
                n133 = local read "Trace Ch Reference"() -> (w285:enum16{"0", "1", "2", "3"})
                n134 = local read "Cursor Windows by Trace"() -> (w276:cluster{"start":dbl, "end":dbl}[])
                n135 = local read "Dual Parameters"() -> (w283:T5)
                n136 = local read "Normalization"() -> (w281:enum16{"None", "Variance", "Sample Num"})
                n137 = local read "Function"() -> (w286:T8)
                n138 = local read "Corr Func"() -> (w282:enum16{"Auto", "Cross"})
                n139 = Unbundle By Name(w279) -> ("File Path List"=w278:path[])
                n140 = Index Array(array=w278) -> (element=w277:path)  [unwired: 1 in]
                n141 = Bundle("Corr Func"=w282, "Normalization"=w281) -> (w280:T36)  [unwired: 1 in]
                n142 = Index Array(array=w276) -> (element=w275:cluster{"start":dbl, "end":dbl})  [unwired: 1 in]
                n143 = call "PowerCorrelation Filename Suggest.vi"("Cursor Window"=w275, "Filepath"=w277, "Correlation"=w280, "Trace Ch Reference"=w285, "Dual Parameters"=w283, "Trace Processing Params"=w284, "Function post process"=w287, "Std Function Parameters"=w288, "Function"=w286) -> ("Analysis Notes"=→"Analysis Notes":string, "Export Name"=w290:string)  [unwired: 1 in]
                n144 = local write "Export Name"(w290) -> ()
              }
            }
          }
          frame "Trace Plot Param" {
            n145 = global read "Plot Globals.vi" "Resp Plots 1"() -> (w299:bool[])
            n146 = call "Set Graph Colors.vi"("Display Flags"=w299) -> ("Current Graph Colors"=w298:u32[])
            n147 = for {
              tunnel: w298 -> [w303] mode=indexing
              i -> [w302]
              n148 = flat-sequence {
                tunnel: w302 -> [w304]
                tunnel: w303 -> [w305]
                frame #0 {
                  n149 = property on="Trace A" class="WFGraph (strict)"("Active Plot"=w304) -> ()  [unwired: 2 in, 2 out]
                  n150 = property on="Trace B" class="WFGraph (strict)"("Active Plot"=w304) -> ()  [unwired: 2 in, 2 out]
                }
                frame #1 {
                  n151 = property on="Trace A" class="WFGraph (strict)"("Plot.Plot Color"=w305) -> ()  [unwired: 2 in, 2 out]
                  n152 = property on="Trace B" class="WFGraph (strict)"("Plot.Plot Color"=w305) -> ()  [unwired: 2 in, 2 out]
                }
              }
            }
            n153 = call "Set Graph Colors.vi"("Display Flags"="Plot Flags 2") -> ("Current Graph Colors"=w296:u32[])
            n154 = for {
              tunnel: w296 -> [w300] mode=indexing
              i -> [w301]
              n155 = property on="Graph 2" class="WFGraph (strict)"("Plot.Plot Color"=w300) -> ()  [unwired: 2 in, 2 out]
              n156 = property on="Graph 2" class="WFGraph (strict)"("Active Plot"=w301) -> ()  [unwired: 2 in, 2 out]
            }
          }
        }
      }
      event "Get File List": Mouse Down {
        n157 = event-data() -> ()  [unwired: 9 out]
        n158 = local read "File Paths"() -> (w310:T9)
        n159 = call "Get File List.vi"("File Paths"=w310, "Display Type"="Display Type") -> ("Okay"=w314:bool, "File Paths"=w311:T9)  [unwired: 4 in, 4 out]
        n160 = case shown="True" w314 {
          tunnel: w313 -> [_ w326]
          tunnel: w311 -> [_ w324]
          tunnel: w308 -> [w319 w323]
          tunnel: [w319 w322] -> w307
          frame False {
          }
          frame True {
            w320 = T21 [enum."Read Data", enum."Variable Update", enum."Plot Traces"] items=["None", "Initialize", "Plot Traces", "Plot Graph2", "Read Data", "Variable Update", "Trace Plot Param"]
            n161 = Unbundle By Name(w324) -> ("File Path List"=w325:path[])
            n162 = for {
              tunnel: w325 -> [w334] mode=indexing
              tunnel: [w335] -> w327 mode=indexing
              n163 = Bundle(w334, "New Data"=TRUE) -> (w335:cluster{path, "New Data":bool})  [unwired: 1 out]
            }
            n164 = for {
              tunnel: w326 -> [w333]
              shift-right: [w331] -> w322
              shift-left: w323 -> [w332]
              tunnel: T20 {"Task"=enum."None", "Argument"=0} ("User Interface Tasks") -> [w330]
              tunnel: w320 -> [w329] mode=indexing
              n165 = Bundle By Name(cluster=w330, "Task"=w329) -> (w328:T20)
              n166 = Generate User Event(user event=w333, event data cluster=w328, error in=w332) -> (error out=w331:errorcluster)  [unwired: 1 in, 1 out]
            }
            n167 = local write "File Path List"(w327) -> ()
            "File Paths" <- w324
          }
        }
      }
      event "Load List File": Mouse Down {
        n168 = event-data() -> ()  [unwired: 9 out]
        n169 = local read "File Paths"() -> (w339:T9)
        n170 = Unbundle By Name(w339) -> ("Listfile Path"=w340:path)
        n171 = call "Read Listfile - high level.vi"("Start Path"=w340) -> ("File Read?"=w344:bool, "File Paths"=w343:path[], "New Start Path"=w342:path)  [unwired: 1 in, 1 out]
        n172 = case shown="True" w344 {
          tunnel: w343 -> [_ w355]
          tunnel: w342 -> [_ w351]
          tunnel: w341 -> [_ w353]
          tunnel: w339 -> [_ w352]
          frame False {
          }
          frame True {
            n173 = for {
              tunnel: w355 -> [w358] mode=indexing
              tunnel: [w356] -> w354 mode=indexing
              n174 = Bundle(w358, "New Data"=TRUE) -> (w356:cluster{path, "New Data":bool})  [unwired: 1 out]
            }
            n175 = Bundle By Name(cluster=w352, "Listfile Path"=w351) -> (w350:T9)
            n176 = local write "File Path List"(w354) -> ()
            n177 = local write "File Paths"(w350) -> ()
            n178 = Generate User Event(user event=w353, event data cluster=T20 {"Task"=enum."Read Data", "Argument"=0} ("User Interface Tasks")) -> ()  [unwired: 2 in, 2 out]
          }
        }
      }
      event "1/2 sample rate": Mouse Down {
        n179 = event-data() -> ()  [unwired: 9 out]
        n180 = Unbundle By Name(w366) -> ("Individual Data Sweeps"=w375:sgl[][], "delta T"=w372:sgl)
        n181 = Unbundle By Name(w367) -> ("Individual Data Sweeps"=w376:sgl[][])
        n182 = Generate User Event(user event=w363, event data cluster=T20 {"Task"=enum."Plot Traces", "Argument"=0} ("User Interface Tasks")) -> ()  [unwired: 2 in, 2 out]
        n183 = Multiply(x=w372, y=sgl 2.0) -> (x*y=w370:sgl)
        n184 = Reciprocal(x=w370) -> (1/x=w369:sgl)
        n185 = for {
          tunnel: w376 -> [w384] mode=indexing
          tunnel: [w383] -> w374 mode=indexing
          tunnel: w375 -> [w382] mode=indexing
          tunnel: [w381] -> w373 mode=indexing
          w379 = 2 ("decimating factor")
          w380 = TRUE
          n186 = call-poly <vilib>:"Decimate (single shot).vi"("averaging"=w380, "decimating factor"=w379, "X"=w384) -> ("Decimated Array"=w383:dbl[])  [unwired: 8 out]
          n187 = call-poly <vilib>:"Decimate (single shot).vi"("averaging"=w380, "decimating factor"=w379, "X"=w382) -> ("Decimated Array"=w381:dbl[])  [unwired: 8 out]
        }
        n188 = Multiply(x=w369, y=sgl 1000.0) -> (x*y=→"samp/sec":sgl)
        n189 = Bundle By Name(cluster=w366, "Individual Data Sweeps"=w373, "delta T"=w370) -> (w364:T19)
        n190 = Bundle By Name(cluster=w367, "Individual Data Sweeps"=w374, "delta T"=w370) -> (w365:T19)
      }
      event "sample rate redux of graph 2": Mouse Up {
        n191 = event-data() -> ()  [unwired: 9 out]
        n192 = Unbundle By Name(w391) -> ("Data"=w397:sgl[][], "dT"=w389:sgl)
        n193 = Generate User Event(user event=w396, event data cluster=T20 {"Task"=enum."Plot Graph2", "Argument"=0} ("User Interface Tasks")) -> ()  [unwired: 2 in, 2 out]
        n194 = Multiply(x=w389, y="redux factor") -> (x*y=w388:sgl)
        n195 = for {
          tunnel: w397 -> [w403] mode=indexing
          tunnel: [w402] -> w386 mode=indexing
          tunnel: "redux factor" -> [w400]
          n196 = call-poly <vilib>:"Decimate (single shot).vi"("averaging"=TRUE, "decimating factor"=w400, "X"=w403) -> ("Decimated Array"=w402:dbl[])  [unwired: 8 out]
        }
        n197 = Multiply(x=w386, y="redux factor") -> (x*y=w385:dbl[][])
        n198 = local write "dF"(w388) -> ()
        n199 = Bundle By Name(cluster=w391, "Data"=w385, "dT"=w388) -> (w390:cluster{"T0":sgl, "dT":sgl, "Data":sgl[][]})
      }
      event "Show All": Mouse Down {
        n200 = event-data() -> ()  [unwired: 9 out]
        n201 = local read "File Path List"() -> (w408:cluster{"FilePath":path, "focus":bool}[])
        n202 = local write "Focus Mode"(FALSE ("Focus Mode")) -> ()
        n203 = local write "Old Focus"(-1 ("Focus")) -> ()
        n204 = for {
          tunnel: w408 -> [w416] mode=indexing
          tunnel: [w414] -> w407 mode=indexing
          n205 = Bundle By Name(cluster=w416, "focus"=TRUE) -> (w414:cluster{"FilePath":path, "focus":bool})
        }
        n206 = local write "File Path List"(w407) -> ()
      }
      event "Focus", "Focus Mode", "File Path List": Value Change {
        n207 = event-data() -> ("NewVal"=→"NewVal 2":variant)  [unwired: 6 out]
        n208 = local read "Focus Mode"() -> (w423:bool)
        n209 = case shown="True" w423 {
          tunnel: w422 -> [_ w432]
          tunnel: w421 -> [w429 w431]
          tunnel: [w429 w430] -> w420
          frame False {
          }
          frame True {
            w433 = T21 [enum."Variable Update", enum."Plot Traces"] items=["None", "Initialize", "Plot Traces", "Plot Graph2", "Read Data", "Variable Update", "Trace Plot Param"]
            n210 = for {
              tunnel: w432 -> [w440]
              shift-right: [w438] -> w430
              shift-left: w431 -> [w439]
              tunnel: T20 {"Task"=enum."None", "Argument"=0} ("User Interface Tasks") -> [w437]
              tunnel: w433 -> [w436] mode=indexing
              n211 = Bundle By Name(cluster=w437, "Task"=w436) -> (w435:T20)
              n212 = Generate User Event(user event=w440, event data cluster=w435, error in=w439) -> (error out=w438:errorcluster)  [unwired: 1 in, 1 out]
            }
          }
        }
        n213 = local write "Assign Cursors In Plot"(TRUE ("Assign Cursors Flag")) -> ()
      }
      event "AP Freq vs Time": Mouse Down {
        n214 = event-data() -> ()  [unwired: 9 out]
        n215 = Generate User Event(user event=w442, event data cluster=T20 {"Task"=enum."Plot Graph2", "Argument"=0} ("User Interface Tasks")) -> ()  [unwired: 2 in, 2 out]
        n216 = call <userlib>:"2D to 1D Trace.vi"("2D Trace In"=w446) -> ("1D Trace Out"=w455:T37)  [unwired: 1 in, 3 out]
        n217 = call <userlib>:"2D to 1D Trace.vi"("2D Trace In"=w445) -> ("1D Trace Out"=w454:T37)  [unwired: 1 in, 3 out]
        n218 = case shown="\"cursors\"" "Window" {
          tunnel: w455 -> [w460 w465]
          tunnel: w454 -> [w459 w463]
          tunnel: [w460 w466] -> w453
          tunnel: [w459 w462] -> w452
          frame "all" {
          }
          frame "cursors" {
            n219 = local read "Focus"() -> (w464:i32)
            n220 = local read "Cursor Windows by Trace"() -> (w467:cluster{"start":dbl, "end":dbl}[])
            n221 = Index Array(array=w467, index=w464) -> (element=w461:cluster{"start":dbl, "end":dbl})
            n222 = call <userlib>:"Trace Subset-general.vi"("Wind (ms)"=w461, "Trace"=w465) -> ("Trace Out"=w466:cluster{"x0":dbl, "dx":dbl, "Data":dbl[]})  [unwired: 2 in]
            n223 = call <userlib>:"Trace Subset-general.vi"("Wind (ms)"=w461, "Trace"=w463) -> ("Trace Out"=w462:cluster{"x0":dbl, "dx":dbl, "Data":dbl[]})  [unwired: 2 in]
          }
        }
        n224 = global read "Display & Avg Globals.vi" "spike trig params"() -> (w447:T38)
        n225 = call "Rate vs Time_2traces.vi"("Mode"=T23."Closest", "Filter Number"=1 ("Element Number"), "AP Freq Mode"="AP Freq Mode", "dx"=sgl 10.0, "spike trig params"=w447, "Trace B"=w452, "Trace A"=w453) -> ("Rate Info"=w444:cluster{"T0":sgl, "Delta T":sgl, "Data":sgl[][]})  [unwired: 2 out]
      }
      event "Do Function": Mouse Down {
        n226 = event-data() -> ()  [unwired: 9 out]
        n227 = local read "Focus Mode"() -> (w483:bool)
        n228 = case shown="\"Trace\"" "Spectrum Source" {
          tunnel: [w685 w696] -> w476
          tunnel: [w684 w696] -> w477
          tunnel: w492 -> [w675 _]
          tunnel: w491 -> [w676 _]
          tunnel: w490 -> [w678 _]
          tunnel: w489 -> [w677 _]
          tunnel: w486 -> [_ w695]
          tunnel: w483 -> [w673 _]
          frame "Trace" {
            n229 = local read "Cursor Windows by Trace"() -> (w674:cluster{"start":dbl, "end":dbl}[])
            n230 = case shown="True" w673 {
              tunnel: [w688 w691] -> w679
              tunnel: [w687 w690] -> w680
              tunnel: w674 -> [w686 w693]
              tunnel: [w686 w692] -> w681
              tunnel: w678 -> [_ w691]
              tunnel: w677 -> [_ w690]
              tunnel: w675 -> [w688 _]
              tunnel: w676 -> [w687 _]
              frame False {
              }
              frame True {
                n231 = local read "Focus"() -> (w689:i32)
                n232 = Array Subset(array=w693, index=w689, length=1) -> (w692:cluster{"start":dbl, "end":dbl}[])
              }
            }
            n233 = call <userlib>:"2D Trace to TraceArray.vi"("2D Trace"=w680) -> ("Trace Array"=w683:cluster{"T0":sgl, "Delta T":sgl, "Data":sgl[]}[])
            n234 = call <userlib>:"2D Trace to TraceArray.vi"("2D Trace"=w679) -> ("Trace Array"=w682:cluster{"T0":sgl, "Delta T":sgl, "Data":sgl[]}[])
            n235 = call <userlib>:"Trace Subset - TraceArray.vi"("Window by Trace"=w681, "Trace Array In"=w683) -> ("Trace Array Out"=w685:cluster{"X0":sgl, "dX":sgl, "Data":sgl[]}[])  [unwired: 2 in, 7 out]
            n236 = call <userlib>:"Trace Subset - TraceArray.vi"("Window by Trace"=w681, "Trace Array In"=w682) -> ("Trace Array Out"=w684:cluster{"X0":sgl, "dX":sgl, "Data":sgl[]}[])  [unwired: 2 in, 7 out]
          }
          frame "Function" {
            n237 = call <userlib>:"2D Trace to TraceArray.vi"("2D Trace"=w695) -> ("Trace Array"=w696:cluster{"T0":sgl, "Delta T":sgl, "Data":sgl[]}[])
          }
        }
        n238 = local read "Trace Processing Params"() -> (w470:T6)
        n239 = Generate User Event(user event=w484, event data cluster=T20 {"Task"=enum."Plot Graph2", "Argument"=0} ("User Interface Tasks")) -> ()  [unwired: 2 in, 2 out]
        n240 = Equal?(x=enum16{"0", "1", "2", "3"}."0", y="Trace Ch Reference") -> (x = y?=w471:bool)
        n241 = Unbundle By Name(w470) -> ("Box Filter Width"=w469:i16)
        n242 = case shown="True" "single chan" {
          tunnel: w477 -> [w494 w497]
          tunnel: w476 -> [w493 w496]
          tunnel: [w494 w495] -> w475
          tunnel: [w493 w495] -> w474
          tunnel: w471 -> [_ w498]
          frame False {
          }
          frame True {
            n243 = Select(t=w497, s=w498, f=w496) -> (s? t:f=w495:cluster{"T0":sgl, "Delta T":sgl, "Data":sgl[]}[])
          }
        }
        n244 = case shown="\"Std Function\", Default" "Function" {
          tunnel: w475 -> [w537 w562 w576 w586 w615 w650 w671]
          tunnel: w474 -> [w536 w561 w575 w585 w614 w649 w670]
          tunnel: [w510 w550 w572 w587 w616 w648 w672] -> w487
          tunnel: w486 -> [w514 _ _ w588 w617 w648 w672]
          tunnel: w483 -> [_ _ _ w589 w618 w647 _]
          tunnel: "window" -> [w521 _ _ w584 _ _ _]
          tunnel: "Trace Ch Reference" -> [w520 w560 w577 w583 w613 _ _]
          tunnel: "Corr Func" -> [_ w549 w571 _ _ _ _]
          tunnel: "Window Size (ms)" -> [_ w548 w570 _ _ _ _]
          tunnel: w469 -> [w499 _ _ _ _ _ _]
          frame "Std Function", Default {
            n245 = local write "Function Units = ms?"(FALSE ("Function Units = ms?")) -> ()
            n246 = call "Dual Channel Analysis-Trace Array"("window"=w521, "Function Parameters"="Std Function Parameters", "Function post process"="Function post process", "Trace Select"=w520, "Trace Array B"=w536, "Trace Array A"=w537) -> ("X Unit"=→"x-axis":string, "Y Unit"=→"y-axis":string, "Individual Functions"=w509:cluster{"X0":sgl, "dX":sgl, "Data":sgl[]}[], "Avg Function"=w502:cluster{"X0":sgl, "Delta X":sgl, "Data":sgl[]}, "Window Constants"=→"Window Constants":cluster{"Eq Noise BW":ext, "Coherent Gain":ext})  [unwired: 1 in]
            n247 = local write "Fourier mode"(TRUE ("Fourier mode")) -> ()
            n248 = call <userlib>:"2D Trace to TraceArray.vi"("2D Trace"=w514) -> ("Trace Array"=w513:cluster{"T0":sgl, "Delta T":sgl, "Data":sgl[]}[])
            n249 = Unbundle By Name("Std Function Parameters") -> ("Function"=w535:u16, "Mag/Phase"=w533:u16)
            n250 = local write "cursor func"(enum16{"2 filter", "+- 10%", "+- 5%", "+-2"}."2 filter" ("cursor func")) -> ()
            n251 = Unbundle By Name(w502) -> ("Delta X"=w529:sgl)
            n252 = Less?(x=w535, y=4) -> (x < y?=w531:bool)
            n253 = Equal To 0?(x=w533) -> (x = 0?=w532:bool)
            n254 = local write "dF"(w529) -> ()
            n255 = local read "Stat Plot"() -> (w505:cluster{dbl[], dbl[]}[])
            n256 = And(x=w531, y=w532) -> (x .and. y?=w530:bool)
            n257 = property on="Stat Plot" class="XYGraph (strict)"() -> ("CrsrList"=w507:T35)  [unwired: 2 in, 2 out]
            n258 = case shown="True" "box filter graph" {
              tunnel: w502 -> [w538 w541]
              tunnel: [w538 w540] -> w501
              tunnel: w499 -> [_ w539]
              frame False {
              }
              frame True {
                n259 = call "Box Average Trace.vi"("Element Number"=w539, "Trace In"=w541) -> ("Trace Out"=w540:cluster{"T0":sgl, "Delta T":sgl, "Data":sgl[]})  [unwired: 1 in, 1 out]
              }
            }
            n260 = case shown="True" w530 {
              tunnel: [0 4] -> w528
              frame False {
              }
              frame True {
              }
            }
            n261 = property on="Graph 2" class="WFGraph (strict)"("YScale.Precision"=w528) -> ()  [unwired: 2 in, 2 out]
            n262 = Initialize Array(TRUE, 1) -> (w524:bool[])
            n263 = Build Array(w501) -> (w512:cluster{"T0":sgl, "Delta T":sgl, "Data":sgl[]}[])
            n264 = call "Add Stat Data Points.vi"("Analysis Transform"="Analysis Transform", "Accumulate Func Plots"="Accumulate Func Plots", "Value"="Value", "Cursor List"=w507, "Individual Functions"=w509, "Stat Plot In"=w505) -> ("Stat Plot Out"=→"Stat Plot":cluster{dbl[], dbl[]}[])  [unwired: 5 in]
            n265 = case shown="False" "Accumulate Func Plots" {
              tunnel: w513 -> [_ w545]
              tunnel: w512 -> [w542 w544]
              tunnel: [w542 w543] -> w511
              frame False {
              }
              frame True {
                n266 = Build Array (concatenate)(w545, w544) -> (w543:cluster{"T0":sgl, "Delta T":sgl, "Data":sgl[]}[])
              }
            }
            n267 = local write "Plot Flags 2"(w524) -> ()
            n268 = call <userlib>:"TraceArray to 2D Trace.vi"("Trace Array"=w511) -> ("2D Trace"=w510:cluster{"X0":sgl, "Delta X":sgl, "Data":sgl[][]})
          }
          frame "Correlation" {
            n269 = call "Correlation-TraceArray.vi"("Normalization"="Normalization", "Correllation Func"="Correllation Func", "Window (ms)"=w548, "Trace Reference"=w560, "Corr Func"=w549, "Trace Array B"=w561, "Trace Array A"=w562) -> ("Correlation Trace"=w564:cluster{"T0":sgl, "Delta T":sgl, "Data":sgl[]})  [unwired: 4 out]
            n270 = Initialize Array(TRUE, 1) -> (w556:bool[])
            n271 = property on="Graph 2" class="WFGraph (strict)"() -> ("X Scale.Range:Maximum"=w554:dbl)  [unwired: 2 in, 2 out]
            n272 = local write "Plot Flags 2"(w556) -> ()
            n273 = call <userlib>:"1D to 2D Trace.vi"("Trace In"=w564) -> ("Trace Out"=w550:cluster{"T0":sgl, "dT":sgl, "Data":sgl[][]})
            n274 = case shown="\"Variance\"" "Normalization" {
              tunnel: ["mV^2" ("y-axis") "unitless" ("y-axis") "mV^2/sample" ("y-axis")] -> w566
              frame "None" {
              }
              frame "Variance" {
              }
              frame "Sample Num" {
              }
            }
            n275 = Negate(x=w554) -> (-x=w553:dbl)
            n276 = local write "y-axis"(w566) -> ()
            n277 = local write "x-axis"("ms" ("x-axis")) -> ()
            n278 = property on="Graph 2" class="WFGraph (strict)"("X Scale.Range:Minimum"=w553) -> ()  [unwired: 2 in, 2 out]
            n279 = property on="Graph 2" class="WFGraph (strict)"("Y Scale.Display Format:Precision"=u8 2 ("Y Precision")) -> ()  [unwired: 2 in, 2 out]
            n280 = local write "Fourier mode"(FALSE ("Fourier mode")) -> ()
            "Function Units = ms?" <- TRUE ("Function Units = ms?")
          }
          frame "Correlation APs" {
            n281 = global read "PowerCorrelation_globals.vi" "AP correl info"() -> (w582:T39)
            n282 = call "AP-Correlation & Interval Hists.vi"("AP correl info"=w582, "Window Size"=w570, "Trace Reference"=w577, "Correlation Function"=w571, "Trace Array B"=w575, "Trace Array A"=w576) -> ("Y-Axis Label"=w581:string, "Ran Value"=→"Ran AP Cor":sgl, "Graphs"=w572:cluster{"T0":sgl, "Delta T":sgl, "Data":sgl[][]})  [unwired: 1 in, 2 out]
            n283 = local write "Function Units = ms?"(TRUE ("Function Units = ms?")) -> ()
            n284 = local write "Fourier mode"(FALSE ("Fourier mode")) -> ()
            n285 = local write "y-axis"(w581) -> ()
            n286 = property on="Graph 2" class="WFGraph (strict)"("Y Scale.Display Format:Precision"=u8 2 ("Y Precision")) -> ()  [unwired: 2 in, 2 out]
            n287 = local write "x-axis"("ms" ("x-axis")) -> ()
          }
          frame "Fourier Trans" {
            n288 = case shown="True" w589 {
              tunnel: w588 -> [w590 _]
              tunnel: [w590 w597] -> w587
              tunnel: w586 -> [_ w607]
              tunnel: w585 -> [_ w606]
              tunnel: w584 -> [_ w598]
              tunnel: w583 -> [_ w594]
              frame False {
              }
              frame True {
                n289 = case shown="\"1\"" w594 {
                  tunnel: w607 -> [w608 _]
                  tunnel: w606 -> [_ w609]
                  tunnel: [w608 w609] -> w605
                  frame "0", Default {
                  }
                  frame "1" {
                  }
                }
                n290 = property on="Graph 2" class="WFGraph (strict)"("XScale.Minimum"=0.0 ("X Minimum")) -> ()  [unwired: 2 in, 2 out]
                n291 = Index Array(array=w605) -> (element=w604:cluster{"T0":sgl, "Delta T":sgl, "Data":sgl[]})  [unwired: 1 in]
                n292 = call "FourierTrans_Reconstruction.vi"("window"=w598, "Amp Coeff Scaling"=enum16{"Reconstruction", "Continous"}."Continous", "Component Num"="Component Num", "Function"=w604) -> ("Reconstruction Function"=w601:cluster{"x0":sgl, "dx":sgl, "array":sgl[]}, "Phase  (degrees)"=w602:cluster{"x0":sgl, "dx":sgl, "array":sgl[]}, "Amp Transform (2x, pos only)"=w603:cluster{"x0":sgl, "dx":sgl, "array":sgl[]})  [unwired: 1 in, 4 out]
                n293 = case shown="\"Reconstruct with FT\"" "Function" {
                  tunnel: w603 -> [w610 _ _]
                  tunnel: w601 -> [_ _ w612]
                  tunnel: [w610 w611 w612] -> w600
                  tunnel: w602 -> [_ w611 _]
                  frame "Fourier Trans - Amp" {
                  }
                  frame "Fourier Trans - Phase" {
                  }
                  frame "Reconstruct with FT" {
                  }
                }
                n294 = local write "Fourier mode"(TRUE ("Fourier mode")) -> ()
                n295 = call <userlib>:"1D to 2D Trace.vi"("Trace In"=w600) -> ("Trace Out"=w597:cluster{"T0":sgl, "dT":sgl, "Data":sgl[][]})
                n296 = Unbundle By Name(w600) -> ("dx"=→"dF":sgl)
              }
            }
          }
          frame "Impulse Resp" {
            n297 = case shown="True" w618 {
              tunnel: [w619 w620] -> w616
              tunnel: w617 -> [w619 _]
              tunnel: w615 -> [_ w634]
              tunnel: w614 -> [_ w633]
              tunnel: w613 -> [_ w621]
              frame False {
              }
              frame True {
                w635 = 0
                n298 = Index Array(array=w634, index=w635) -> (element=w623:cluster{"T0":sgl, "Delta T":sgl, "Data":sgl[]})
                n299 = Index Array(array=w633, index=w635) -> (element=w622:cluster{"T0":sgl, "Delta T":sgl, "Data":sgl[]})
                n300 = case shown="\"0\", Default" w621 {
                  tunnel: w623 -> [w637 w639]
                  tunnel: w622 -> [w636 w638]
                  tunnel: [w637 w638] -> w632
                  tunnel: [w636 w639] -> w631
                  frame "0", Default {
                  }
                  frame "1" {
                  }
                }
                n301 = Unbundle By Name(w631) -> ("Data"=w629:sgl[], "Delta T"=w627:sgl)
                n302 = Unbundle By Name(w632) -> ("Data"=w630:sgl[])
                n303 = case shown="True" TRUE {
                  tunnel: w630 -> [w643 w646]
                  tunnel: w629 -> [w642 w645]
                  tunnel: [w640 w644] -> w628
                  tunnel: w627 -> [w641 _]
                  frame False {
                    n304 = call <vilib>:"Transfer Function.vi"("dt"=w641, "Response Signal"=w642, "Stimulus Signal"=w643) -> ("Frequency Response Phase (radians)"=w640:dbl[])  [unwired: 2 out]
                  }
                  frame True {
                    n305 = call <vilib>:"Impulse Response Function.vi"("Signal Y Response"=w645, "Signal X Stimulus"=w646) -> ("Impulse Response"=w644:dbl[])
                  }
                }
                n306 = Bundle(0, "Delta T"=w627, "Impulse Response"=w628) -> (w625:T40)  [unwired: 1 out]
                n307 = call <userlib>:"1D to 2D Trace.vi"("Trace In"=w625) -> ("Trace Out"=w620:cluster{"T0":sgl, "dT":sgl, "Data":sgl[][]})
              }
            }
          }
          frame "CV's" {
            n308 = case shown="True" w647 {
              tunnel: w650 -> [_ w652]
              tunnel: w649 -> [_ w651]
              frame False {
              }
              frame True {
                w667 = 0
                n309 = Index Array(array=w651, index=w667) -> (element=w666:cluster{"T0":sgl, "Delta T":sgl, "Data":sgl[]})
                n310 = Index Array(array=w652, index=w667) -> (element=w665:cluster{"T0":sgl, "Delta T":sgl, "Data":sgl[]})
                n311 = call "Get Spike Times.vi"("Trace"=w665) -> ("Spike Times"=w664:sgl[])  [unwired: 2 in, 8 out]
                n312 = call "Get Spike Times.vi"("Trace"=w666) -> ("Spike Times"=w663:sgl[])  [unwired: 2 in, 8 out]
                n313 = call <userlib>:"Difference Array.vi"("Array"=w664) -> ("Difference Array"=w662:sgl[])  [unwired: 1 in, 5 out]
                n314 = call <userlib>:"Difference Array.vi"("Array"=w663) -> ("Difference Array"=w661:sgl[])  [unwired: 1 in, 5 out]
                n315 = call <vilib>:"Std Deviation and Variance.vi"("X"=w662, "Weighting (Sample)"=enum16{"Sample", "Population"}."Population") -> ("mean"=w656:dbl, "standard deviation"=w657:dbl)  [unwired: 1 out]
                n316 = call <vilib>:"Std Deviation and Variance.vi"("X"=w661, "Weighting (Sample)"=enum16{"Sample", "Population"}."Population") -> ("mean"=w659:dbl, "standard deviation"=w660:dbl)  [unwired: 1 out]
                n317 = Divide(x=w657, y=w656) -> (x/y=→"CV A":dbl)
                n318 = Divide(x=w660, y=w659) -> (x/y=→"CV B":dbl)
              }
            }
          }
          frame "SD's" {
            n319 = call "Standard Deviation_Trace Array.vi"("Trace Array"=w671) -> ("Std Dev"=→"SD A":sgl)  [unwired: 10 out]
            n320 = call "Standard Deviation_Trace Array.vi"("Trace Array"=w670) -> ("Std Dev"=→"SD B":sgl)  [unwired: 10 out]
          }
        }
      }
      event "Function post process", "Function", "Std Function Parameters", "Trace Ch Reference": Value Change {
        n321 = event-data() -> ()  [unwired: 7 out]
        n322 = Generate User Event(user event=w698, event data cluster=T20 {"Task"=enum."Variable Update", "Argument"=0} ("User Interface Tasks")) -> ()  [unwired: 2 in, 2 out]
      }
      event "Time Course": Mouse Down {
        n323 = event-data() -> ()  [unwired: 9 out]
        n324 = local read "Focus Mode"() -> (w709:bool)
        n325 = case shown="True" w709 {
          tunnel: w708 -> [_ w714]
          tunnel: w707 -> [_ w713]
          frame False {
          }
          frame True {
            n326 = local read "Cursor Windows by Trace"() -> (w722:cluster{"start":dbl, "end":dbl}[])
            n327 = local read "Focus"() -> (w721:i32)
            n328 = Index Array(array=w722, index=w721) -> (element=w712:cluster{"start":dbl, "end":dbl})
            n329 = local read "Window Size (ms)"() -> (w730:sgl)
            n330 = call <userlib>:"2D to 1D Trace.vi"("2D Trace In"=w714) -> ("1D Trace Out"=w717:T37)  [unwired: 1 in, 3 out]
            n331 = call <userlib>:"2D to 1D Trace.vi"("2D Trace In"=w713) -> ("1D Trace Out"=w720:T37)  [unwired: 1 in, 3 out]
            n332 = local read "Std Function Parameters"() -> (w735:T18)
            n333 = local read "Normalization"() -> (w729:enum16{"None", "Variance", "Sample Num"})
            n334 = local read "Corr Func"() -> (w731:enum16{"Auto", "Cross"})
            n335 = local read "Trace Ch Reference"() -> (w738:enum16{"0", "1", "2", "3"})
            n336 = global read "PowerCorrelation_globals.vi" "AP correl info"() -> (w723:T39)
            n337 = local read "Function post process"() -> (w715:T11)
            n338 = call <userlib>:"Trace Subset-general.vi"("Wind (ms)"=w712, "Trace"=w717) -> ("Trace Out"=w716:cluster{"x0":dbl, "dx":dbl, "Data":dbl[]})  [unwired: 2 in]
            n339 = call <userlib>:"Trace Subset-general.vi"("Wind (ms)"=w712, "Trace"=w720) -> ("Trace Out"=w718:cluster{"x0":dbl, "dx":dbl, "Data":dbl[]})  [unwired: 2 in]
            n340 = Bundle("Corr Func"=w731, "Window Size (ms)"=w730, "Normalization"=w729) -> (w728:T41)  [unwired: 1 out]
            n341 = global read "Display & Avg Globals.vi" "spike trig params"() -> (w724:T38)
            n342 = local read "window"() -> (w736:T17)
            n343 = call "Time Course Spectrum.vi"("Trace A"=w716, "Trace B"=w718, "Function"="Function", "Trace Select"=w738, "Raw Data Function Parameters"=w735, "AP correl info"=w723, "Time Course Increment (ms)"="Time Course Increment", "Function post process"=w715, "Moving Win Size (ms)"="Time Course Window", "window"=w736, "Correlation Parameters"=w728, "spike trig params"=w724) -> ("Time Course Data"=w737:sgl[][], "x axis info out"=w727:cluster{"x0":dbl, "dx":dbl}, "y axis info out"=w726:cluster{"y0":dbl, "dy":dbl})  [unwired: 3 in, 2 out]
            n344 = Unbundle By Name(w726) -> ("dy"=w725:dbl)
            n345 = local write "dF"(w725) -> ()
            n346 = case shown="\"1\"" "Time Course Focus" {
              tunnel: w737 -> [w741 w744]
              tunnel: w727 -> [w740 w743]
              tunnel: w726 -> [w739 w742]
              frame "1" {
                n347 = property on="Time Course Function" class="IntGraph (strict)"("X Scale.Offset and Multiplier"=w740) -> ()  [unwired: 2 in, 2 out]
                n348 = property on="Time Course Function" class="IntGraph (strict)"("Y Scale.Offset and Multiplier"=w739) -> ()  [unwired: 2 in, 2 out]
                "Time Course 1" <- w741
              }
              frame "2" {
                n349 = property on="Time Course 2" class="IntGraph (strict)"("X Scale.Offset and Multiplier"=w743) -> ()  [unwired: 2 in, 2 out]
                n350 = property on="Time Course 2" class="IntGraph (strict)"("Y Scale.Offset and Multiplier"=w742) -> ()  [unwired: 2 in, 2 out]
                "Time Course 2" <- w744
              }
            }
          }
        }
      }
      event "Add Datum", "Init Data", "Graph Data": Value Change {
        n351 = event-data() -> ()  [unwired: 7 out]
        n352 = case shown="True" "Graph Data" {
          frame False {
          }
          frame True {
            n353 = Greater?(x="Graph Mode", y=enum16{"Points", "Max", "Min"}."Points" ("Graph Mode")) -> (0:w755:bool)
            n354 = case shown="True" w755 {
              tunnel: "Graph Mode" -> [_ w767]
              frame False {
                n355 = local read "x"() -> (w761:sgl[])
                n356 = Index Array(array=w761, index=1) -> (element=w762:sgl)
                n357 = Index Array(array=w761, index=0) -> (element=w763:sgl)
                n358 = local read "Data"() -> (w764:sgl[])
                n359 = Subtract(x=w762, y=w763) -> (x-y=w759:sgl)
                n360 = Build Array(w764) -> (w765:sgl[][])
                n361 = Bundle(w763, w759, w765) -> (w760:cluster{sgl, sgl, sgl[][]})  [unwired: 1 out]
                n362 = local write "Graph 2"(w760) -> ()
              }
              frame True {
                n363 = case shown="\"Max\"" w767 {
                  tunnel: [enum16{"Max", "Min"}."Max" ("Mode") enum16{"Max", "Min"}."Max" ("Mode") enum16{"Max", "Min"}."Min" ("Mode")] -> w766
                  frame "Points" {
                  }
                  frame "Max" {
                  }
                  frame "Min" {
                  }
                }
                n364 = local read "Time Course Focus"() -> (w768:enum16{"1", "2"})
                n365 = property on="Time Course 1" class="IntGraph (strict)"() -> ("Old Cursor List"=w769:T42)  [unwired: 2 in, 2 out]
                n366 = local read "Time Course 1"() -> (w772:sgl[][])
                n367 = case shown="\"2\"" w768 {
                  tunnel: [w784 w785] -> w774
                  frame "1" {
                    n368 = local read "Time Course 1"() -> (w784:sgl[][])
                  }
                  frame "2" {
                    n369 = local read "Time Course 2"() -> (w785:sgl[][])
                  }
                }
                n370 = call "Cursor Positions_IntensityGraph.vi"("Cursor List (old)"=w769) -> ("Coords0"=w775:cluster{"x":sgl, "y":sgl}, "indices1"=w771:cluster{"row":i32, "col":i32}, "indices0"=w770:cluster{"row":i32, "col":i32})  [unwired: 1 in, 5 out]
                n371 = call <userlib>:"Subset_2DArray.vi"("Mode"=w766, "indices end"=w771, "indices start"=w770, "2D Array"=w772) -> ("Index Array"=w773:cluster{"row":i32, "col":i32}[])  [unwired: 5 out]
                n372 = Unbundle By Name(w775) -> ("x"=w776:sgl)
                n373 = for {
                  tunnel: w773 -> [w789] mode=indexing
                  tunnel: w774 -> [w788]
                  tunnel: [w787] -> w777 mode=indexing
                  n374 = case shown="\"y\"" "Coord" {
                    tunnel: [w793 w799] -> w787
                    tunnel: w788 -> [_ w798]
                    tunnel: w789 -> [w796 w797]
                    frame "y" {
                      n375 = property on="Time Course 1" class="IntGraph (strict)"() -> ("Y Scale.Offset and Multiplier"=w792:T43)  [unwired: 2 in, 2 out]
                      n376 = Unbundle By Name(w792) -> ("Offset"=w791:dbl, "Multiplier"=w790:dbl)
                      n377 = Unbundle By Name(w796) -> ("row"=w795:i32)
                      n378 = Multiply(x=w790, y=w795) -> (x*y=w794:dbl)
                      n379 = Add(x=w791, y=w794) -> (x+y=w793:dbl)
                    }
                    frame "z" {
                      n380 = Unbundle By Name(w797) -> ("col"=w800:i32, "row"=w801:i32)
                      n381 = Index Array(array=w798, index (row)=w800, index (col)=w801) -> (element=w799:sgl)
                    }
                  }
                }
                n382 = property on="Time Course 1" class="IntGraph (strict)"() -> ("X Scale.Offset and Multiplier:Multiplier"=w779:dbl)  [unwired: 2 in, 2 out]
                n383 = Build Array(w777) -> (w778:dbl[][])
                n384 = Bundle("x"=w776, "XScale.Multiplier"=w779, w778) -> (w780:T44)  [unwired: 1 out]
                n385 = local write "Graph 2"(w780) -> ()
              }
            }
          }
        }
        n386 = case shown="True" "Add Datum" {
          frame False {
          }
          frame True {
            n387 = local read "Time Course Focus"() -> (w813:enum16{"1", "2"})
            n388 = case shown="\"1\"" w813 {
              tunnel: [w814 w815] -> w812
              frame "1" {
                n389 = local read "Time Course 1"() -> (w814:sgl[][])
              }
              frame "2" {
                n390 = local read "Time Course 2"() -> (w815:sgl[][])
              }
            }
            n391 = property on="Time Course 1" class="IntGraph (strict)"() -> ("Cursor.Cursor Index"=w803:i32)  [unwired: 2 in, 2 out]
            n392 = property on="Time Course 1" class="IntGraph (strict)"() -> ("Cursor.Cursor Plot"=w804:i32)  [unwired: 2 in, 2 out]
            n393 = Index Array(array=w812, index (row)=w803, index (col)=w804) -> (element=w810:sgl)
            n394 = local read "x"() -> (w806:sgl[])
            n395 = local read "y"() -> (w805:sgl[])
            n396 = local read "Data"() -> (w811:sgl[])
            n397 = Build Array (concatenate)(w805, w804) -> (w807:sgl[])
            n398 = Build Array (concatenate)(w811, w810) -> (w809:sgl[])
            n399 = Build Array (concatenate)(w806, w803) -> (w808:sgl[])
            n400 = local write "Data"(w809) -> ()
            n401 = local write "x"(w808) -> ()
            n402 = local write "y"(w807) -> ()
          }
        }
        n403 = case shown="True" "Init Data" {
          frame False {
          }
          frame True {
            w802 = sgl[] []
            "Data" <- w802
            "x" <- w802
            "y" <- w802
          }
        }
      }
      event "zoom", "expand": Mouse Down {
        # "only applies to graph 2!!!"
        n404 = event-data() -> ()  [unwired: 9 out]
        n405 = property on="Graph 2" class="WFGraph (strict)"() -> ("X Scale.Range:Maximum"=w822:dbl)  [unwired: 2 in, 2 out]
        n406 = case shown="False" "expand" {
          tunnel: w822 -> [w828 w832]
          tunnel: [w827 w831] -> w821
          tunnel: 2.0 ("y") -> [w829 w830]
          frame False {
            n407 = Divide(x=w828, y=w829) -> (x/y=w827:dbl)
          }
          frame True {
            n408 = Multiply(x=w832, y=w830) -> (x*y=w831:dbl)
          }
        }
        n409 = case shown="False" "Fourier mode" {
          tunnel: w821 -> [w834 _]
          frame False {
            n410 = Negate(x=w834) -> (-x=w833:dbl)
            n411 = property on="Graph 2" class="WFGraph (strict)"("X Scale.Range:Minimum"=w833) -> ()  [unwired: 2 in, 2 out]
          }
          frame True {
          }
        }
        n412 = property on="Graph 2" class="WFGraph (strict)"("X Scale.Range:Maximum"=w821) -> ()  [unwired: 2 in, 2 out]
      }
      event "scale": Mouse Up {
        n413 = event-data() -> ()  [unwired: 9 out]
        n414 = case shown="\"Trace Ch\"" "Func Mode" {
          tunnel: w844 -> [w854 w878]
          tunnel: w843 -> [w853 w877]
          tunnel: [w852 w875] -> w842
          tunnel: [w851 w876] -> w841
          tunnel: "scale" -> [w850 w874]
          tunnel: "Offset/Sc/Ph" -> [w848 w873]
          frame "Trace #", Default {
            n415 = call <userlib>:"2D Trace to TraceArray.vi"("2D Trace"=w854) -> ("Trace Array"=w860:cluster{"T0":sgl, "Delta T":sgl, "Data":sgl[]}[])
            n416 = call <userlib>:"2D Trace to TraceArray.vi"("2D Trace"=w853) -> ("Trace Array"=w858:cluster{"T0":sgl, "Delta T":sgl, "Data":sgl[]}[])
            n417 = Index Array(array=w858, index="Trace #") -> (element=w861:cluster{"T0":sgl, "Delta T":sgl, "Data":sgl[]})
            n418 = Index Array(array=w860, index="Trace #") -> (element=w862:cluster{"T0":sgl, "Delta T":sgl, "Data":sgl[]})
            n419 = case shown="True" w850 {
              tunnel: w862 -> [w867 w872]
              tunnel: w861 -> [w864 w871]
              tunnel: w848 -> [w863 w870]
              tunnel: [w866 w869] -> w859
              tunnel: [w865 w868] -> w857
              frame False {
                n420 = call <userlib>:"Shift Trace.vi"("Shift (dt units)"=w863, "Trace In"=w867) -> ("Trace Out"=w866:cluster{"T0":sgl, "dT":sgl, "Data":sgl[]})  [unwired: 3 out]
                n421 = call <userlib>:"Shift Trace.vi"("Shift (dt units)"=w863, "Trace In"=w864) -> ("Trace Out"=w865:cluster{"T0":sgl, "dT":sgl, "Data":sgl[]})  [unwired: 3 out]
              }
              frame True {
                n422 = call <userlib>:"Scale Trace.vi"("Scale Factor"=w870, "Trace In"=w872) -> ("Scaled Trace"=w869:cluster{"T0":sgl, "Delta T":sgl, "Data":sgl[]})  [unwired: 9 out]
                n423 = call <userlib>:"Scale Trace.vi"("Scale Factor"=w870, "Trace In"=w871) -> ("Scaled Trace"=w868:cluster{"T0":sgl, "Delta T":sgl, "Data":sgl[]})  [unwired: 9 out]
              }
            }
            n424 = Replace Array Subset(array=w860, new element=w859, index="Trace #") -> (w855:cluster{"T0":sgl, "Delta T":sgl, "Data":sgl[]}[])
            n425 = Replace Array Subset(array=w858, new element=w857, index="Trace #") -> (w856:cluster{"T0":sgl, "Delta T":sgl, "Data":sgl[]}[])
            n426 = call <userlib>:"TraceArray to 2D Trace.vi"("Trace Array"=w855) -> ("2D Trace"=w852:cluster{"X0":sgl, "Delta X":sgl, "Data":sgl[][]})
            n427 = call <userlib>:"TraceArray to 2D Trace.vi"("Trace Array"=w856) -> ("2D Trace"=w851:cluster{"X0":sgl, "Delta X":sgl, "Data":sgl[][]})
          }
          frame "Trace Ch" {
            n428 = local read "Trace Ch Reference"() -> (w883:enum16{"0", "1", "2", "3"})
            n429 = case shown="\"0\", Default" w883 {
              tunnel: [w898 w899] -> w882
              tunnel: w878 -> [w898 _]
              tunnel: w877 -> [_ w899]
              frame "0", Default {
              }
              frame "1" {
              }
            }
            n430 = call <userlib>:"2D Trace to TraceArray.vi"("2D Trace"=w882) -> ("Trace Array"=w881:cluster{"T0":sgl, "Delta T":sgl, "Data":sgl[]}[])
            n431 = for {
              tunnel: w881 -> [w891] mode=indexing
              tunnel: [w890] -> w880 mode=indexing
              tunnel: w874 -> [w889]
              tunnel: w873 -> [w888]
              n432 = case shown="True" w889 {
                tunnel: w888 -> [w892 w897]
                tunnel: w891 -> [w894 w896]
                tunnel: [w893 w895] -> w890
                frame False {
                  n433 = call <userlib>:"Shift Trace.vi"("Shift (dt units)"=w892, "Trace In"=w894) -> ("Trace Out"=w893:cluster{"T0":sgl, "dT":sgl, "Data":sgl[]})  [unwired: 3 out]
                }
                frame True {
                  n434 = call <userlib>:"Scale Trace.vi"("Scale Factor"=w897, "Trace In"=w896) -> ("Scaled Trace"=w895:cluster{"T0":sgl, "Delta T":sgl, "Data":sgl[]})  [unwired: 9 out]
                }
              }
            }
            n435 = call <userlib>:"TraceArray to 2D Trace.vi"("Trace Array"=w880) -> ("2D Trace"=w879:cluster{"X0":sgl, "Delta X":sgl, "Data":sgl[][]})
            n436 = case shown="\"0\", Default" w883 {
              tunnel: w879 -> [w885 w887]
              tunnel: [w885 w886] -> w875
              tunnel: w878 -> [_ w886]
              tunnel: w877 -> [w884 _]
              tunnel: [w884 w887] -> w876
              frame "0", Default {
              }
              frame "1" {
              }
            }
          }
        }
        n437 = Generate User Event(user event=w840, event data cluster=T20 {"Task"=enum."Plot Traces", "Argument"=0} ("User Interface Tasks")) -> ()  [unwired: 2 in, 2 out]
      }
      event "Traces\nmV to uV": Mouse Up {
        n438 = event-data() -> ()  [unwired: 9 out]
        n439 = local read "Func Mode"() -> (w900:enum16{"Trace #", "Trace Ch"})
        n440 = case shown="\"Trace Ch\"" w900 {
          tunnel: w909 -> [w917 w931]
          tunnel: w908 -> [w916 w930]
          tunnel: [w915 w928] -> w907
          tunnel: [w914 w929] -> w906
          tunnel: sgl 1000.0 ("Offset/Sc/Ph 2") -> [w912 w927]
          frame "Trace #", Default {
            n441 = call <userlib>:"2D Trace to TraceArray.vi"("2D Trace"=w917) -> ("Trace Array"=w923:cluster{"T0":sgl, "Delta T":sgl, "Data":sgl[]}[])
            n442 = call <userlib>:"2D Trace to TraceArray.vi"("2D Trace"=w916) -> ("Trace Array"=w921:cluster{"T0":sgl, "Delta T":sgl, "Data":sgl[]}[])
            n443 = Index Array(array=w921, index="Trace # 2") -> (element=w924:cluster{"T0":sgl, "Delta T":sgl, "Data":sgl[]})
            n444 = Index Array(array=w923, index="Trace # 2") -> (element=w925:cluster{"T0":sgl, "Delta T":sgl, "Data":sgl[]})
            n445 = call <userlib>:"Scale Trace.vi"("Scale Factor"=w912, "Trace In"=w925) -> ("Scaled Trace"=w922:cluster{"T0":sgl, "Delta T":sgl, "Data":sgl[]})  [unwired: 9 out]
            n446 = call <userlib>:"Scale Trace.vi"("Scale Factor"=w912, "Trace In"=w924) -> ("Scaled Trace"=w920:cluster{"T0":sgl, "Delta T":sgl, "Data":sgl[]})  [unwired: 9 out]
            n447 = Replace Array Subset(array=w923, new element=w922, index="Trace # 2") -> (w918:cluster{"T0":sgl, "Delta T":sgl, "Data":sgl[]}[])
            n448 = Replace Array Subset(array=w921, new element=w920, index="Trace # 2") -> (w919:cluster{"T0":sgl, "Delta T":sgl, "Data":sgl[]}[])
            n449 = call <userlib>:"TraceArray to 2D Trace.vi"("Trace Array"=w918) -> ("2D Trace"=w915:cluster{"X0":sgl, "Delta X":sgl, "Data":sgl[][]})
            n450 = call <userlib>:"TraceArray to 2D Trace.vi"("Trace Array"=w919) -> ("2D Trace"=w914:cluster{"X0":sgl, "Delta X":sgl, "Data":sgl[][]})
          }
          frame "Trace Ch" {
            n451 = local read "Trace Ch Reference"() -> (w936:enum16{"0", "1", "2", "3"})
            n452 = case shown="\"0\", Default" w936 {
              tunnel: [w946 w947] -> w935
              tunnel: w931 -> [w946 _]
              tunnel: w930 -> [_ w947]
              frame "0", Default {
              }
              frame "1" {
              }
            }
            n453 = call <userlib>:"2D Trace to TraceArray.vi"("2D Trace"=w935) -> ("Trace Array"=w934:cluster{"T0":sgl, "Delta T":sgl, "Data":sgl[]}[])
            n454 = for {
              tunnel: w934 -> [w945] mode=indexing
              tunnel: [w944] -> w933 mode=indexing
              tunnel: w927 -> [w943]
              n455 = call <userlib>:"Scale Trace.vi"("Scale Factor"=w943, "Trace In"=w945) -> ("Scaled Trace"=w944:cluster{"T0":sgl, "Delta T":sgl, "Data":sgl[]})  [unwired: 9 out]
            }
            n456 = call <userlib>:"TraceArray to 2D Trace.vi"("Trace Array"=w933) -> ("2D Trace"=w932:cluster{"X0":sgl, "Delta X":sgl, "Data":sgl[][]})
            n457 = case shown="\"1\"" w936 {
              tunnel: w932 -> [w939 w942]
              tunnel: [w939 w941] -> w928
              tunnel: w931 -> [_ w941]
              tunnel: w930 -> [w938 _]
              tunnel: [w938 w942] -> w929
              tunnel: "uV" ("Trace B units") -> [w937 w940]
              frame "0", Default {
                n458 = local write "Trace A units"(w937) -> ()
              }
              frame "1" {
                n459 = local write "Trace B units"(w940) -> ()
              }
            }
          }
        }
        n460 = Generate User Event(user event=w905, event data cluster=T20 {"Task"=enum."Plot Traces", "Argument"=0} ("User Interface Tasks")) -> ()  [unwired: 2 in, 2 out]
      }
      event "Filter": Mouse Down {
        w953 = T21 [enum."Variable Update", enum."Plot Traces"] items=["None", "Initialize", "Plot Traces", "Plot Graph2", "Read Data", "Variable Update", "Trace Plot Param"]
        n461 = event-data() -> ()  [unwired: 9 out]
        n462 = local write "Old Focus"(-1 ("Old Focus")) -> ()
        n463 = Bundle("Ref Wind Start (ms)"=0.0, "Ref Wind End (ms)"=1000000.0) -> (w957:T45)  [unwired: 1 in]
        n464 = call <userlib>:"Offset 2D Trace.vi"("Ref Wind (ms)"=w957, "Traces In"=w963) -> ("Offset Traces Out"=w955:cluster{"T0":sgl, "Delta T":sgl, "Data":sgl[][]})  [unwired: 2 in, 7 out]
        n465 = call <userlib>:"Offset 2D Trace.vi"("Ref Wind (ms)"=w957, "Traces In"=w964) -> ("Offset Traces Out"=w956:cluster{"T0":sgl, "Delta T":sgl, "Data":sgl[][]})  [unwired: 2 in, 7 out]
        n466 = case shown="False" FALSE {
          tunnel: [w979 w991] -> w962
          tunnel: [w975 w990] -> w961
          tunnel: w956 -> [w982 w989]
          tunnel: w955 -> [w978 w987]
          frame False {
            n467 = Build Array(w982) -> (w981:T46)
            n468 = Build Array(w978) -> (w977:T46)
            n469 = call "Composite Array Filter.vi"("Trace Processing Params"="Trace Processing Params", "Composite Array In"=w981) -> ("Composite Array Out"=w980:cluster{"T0":sgl, "dT":sgl, "Data":sgl[][]}[])  [unwired: 5 in]
            n470 = call "Composite Array Filter.vi"("Trace Processing Params"="Trace Processing Params", "Composite Array In"=w977) -> ("Composite Array Out"=w976:cluster{"T0":sgl, "dT":sgl, "Data":sgl[][]}[])  [unwired: 5 in]
            n471 = Index Array(array=w980) -> (element=w979:cluster{"T0":sgl, "dT":sgl, "Data":sgl[][]})  [unwired: 1 in]
            n472 = Index Array(array=w976) -> (element=w975:cluster{"T0":sgl, "dT":sgl, "Data":sgl[][]})  [unwired: 1 in]
          }
          frame True {
            n473 = call <userlib>:"2D Trace to TraceArray.vi"("2D Trace"=w989) -> ("Trace Array"=w988:cluster{"T0":sgl, "Delta T":sgl, "Data":sgl[]}[])
            n474 = call <userlib>:"2D Trace to TraceArray.vi"("2D Trace"=w987) -> ("Trace Array"=w986:cluster{"T0":sgl, "Delta T":sgl, "Data":sgl[]}[])
            n475 = for {
              tunnel: w988 -> [w997] mode=indexing
              tunnel: w986 -> [w996] mode=indexing
              tunnel: [w995] -> w985
              tunnel: [w994] -> w984 mode=indexing
              tunnel: [w993] -> w983 mode=indexing
              w992 = TRUE ("Cut to Original Length")
              n476 = call "Filter Trace.vi"("Cut to Original Length"=w992, "Trace In"=w996) -> ("Message"=w995:string, "Trace Out"=w993:cluster{"x0":sgl, "dx":sgl, "Data":sgl[]})  [unwired: 5 in, 3 out]
              n477 = call "Filter Trace.vi"("Cut to Original Length"=w992, "Trace In"=w997) -> ("Trace Out"=w994:cluster{"x0":sgl, "dx":sgl, "Data":sgl[]})  [unwired: 5 in, 4 out]
            }
            n478 = local write "Message"(w985) -> ()
            n479 = call <userlib>:"TraceArray to 2D Trace.vi"("Trace Array"=w984) -> ("2D Trace"=w991:cluster{"X0":sgl, "Delta X":sgl, "Data":sgl[][]})
            n480 = call <userlib>:"TraceArray to 2D Trace.vi"("Trace Array"=w983) -> ("2D Trace"=w990:cluster{"X0":sgl, "Delta X":sgl, "Data":sgl[][]})
          }
        }
        n481 = for {
          tunnel: w951 -> [w973]
          shift-right: [w971] -> w949
          shift-left: w950 -> [w972]
          tunnel: T20 {"Task"=enum."None", "Argument"=0} ("User Interface Tasks") -> [w970]
          tunnel: w953 -> [w969] mode=indexing
          n482 = Bundle By Name(cluster=w970, "Task"=w969) -> (w968:T20)
          n483 = Generate User Event(user event=w973, event data cluster=w968, error in=w972) -> (error out=w971:errorcluster)  [unwired: 1 in, 1 out]
        }
      }
      event "Trace Processing Params": Value Change {
        n484 = event-data() -> ()  [unwired: 7 out]
      }
      event "Filter Function": Mouse Down {
        # "Put cursors in correct place"
        n485 = event-data() -> ()  [unwired: 9 out]
        n486 = local read "Graph 2"() -> (w1014:cluster{"T0":sgl, "delta T":sgl, sgl[][]})
        n487 = Generate User Event(user event=w1005, event data cluster=T20 {"Task"=enum."Plot Graph2", "Argument"=0} ("User Interface Tasks")) -> ()  [unwired: 2 in, 2 out]
        n488 = call <userlib>:"2D Trace to TraceArray.vi"("2D Trace"=w1014) -> ("Trace Array"=w1013:cluster{"T0":sgl, "Delta T":sgl, "Data":sgl[]}[])
        n489 = Index Array(array=w1013, index=0) -> (element=w1015:cluster{"T0":sgl, "Delta T":sgl, "Data":sgl[]})
        n490 = local read "Function Units = ms?"() -> (w1009:bool)
        n491 = call "Filter Trace.vi"("trace in ms?"=w1009, "Cut to Original Length"=TRUE, "band type"=T24."Lowpass" ("filter type"), "Low Cutoff"="Cutoff (cyc/Hz or Hz)", "Filter Type"=enum16{"none", "FIR", "Butterworth"}."FIR", "Trace In"=w1015) -> ("Trace Out"=w1012:cluster{"x0":sgl, "dx":sgl, "Data":sgl[]})  [unwired: 1 in, 4 out]
        n492 = Replace Array Subset(array=w1013, new element=w1012, index=0) -> (w1010:cluster{"T0":sgl, "Delta T":sgl, "Data":sgl[]}[])
        n493 = call <userlib>:"TraceArray to 2D Trace.vi"("Trace Array"=w1010) -> ("2D Trace"=w1007:cluster{"X0":sgl, "Delta X":sgl, "Data":sgl[][]})
        n494 = stacked-sequence {
          tunnel: w1007 -> [_ _ _ _ _ _]
          frame #0 {
            n495 = property on="Graph 2" class="WFGraph (strict)"("Active Cursor"=u32 0) -> ()  [unwired: 2 in, 2 out]
          }
          frame #1 {
            n496 = property on="Graph 2" class="WFGraph (strict)"("Cursor.Cursor Lock Style"=u32 0 ("Cursor Locked")) -> ()  [unwired: 2 in, 2 out]
          }
          frame #2 {
            n497 = local read "Graph 2 - cursor 0 x"() -> (w1026:sgl)
            n498 = property on="Graph 2" class="WFGraph (strict)"("Cursor.Cursor Position:Cursor X"=w1026) -> ()  [unwired: 2 in, 2 out]
          }
          frame #3 {
            n499 = property on="Graph 2" class="WFGraph (strict)"("Active Cursor"=u32 1) -> ()  [unwired: 2 in, 2 out]
          }
          frame #4 {
            n500 = property on="Graph 2" class="WFGraph (strict)"("Cursor.Cursor Lock Style"=u32 0 ("Cursor Locked")) -> ()  [unwired: 2 in, 2 out]
          }
          frame #5 {
            n501 = local read "Graph 2 - cursor 1 x"() -> (w1029:sgl)
            n502 = property on="Graph 2" class="WFGraph (strict)"("Cursor.Cursor Position:Cursor X"=w1029) -> ()  [unwired: 2 in, 2 out]
          }
        }
      }
      event "Offset Traces": Mouse Down {
        w1033 = T21 [enum."Variable Update", enum."Plot Traces"] items=["None", "Initialize", "Plot Traces", "Plot Graph2", "Read Data", "Variable Update", "Trace Plot Param"]
        # "offset traces will offset based on individual cursor locations in focus mode.  only cursor set 0 when not in focus mode"
        n503 = event-data() -> ()  [unwired: 9 out]
        n504 = local read "Focus Mode"() -> (w1045:bool)
        n505 = case shown="True" w1045 {
          tunnel: [0 ("Focus") w1055] -> w1044
          frame False {
          }
          frame True {
            n506 = local read "Focus"() -> (w1055:i32)
          }
        }
        n507 = local read "Offset/Sc/Ph"() -> (w1042:sgl)
        n508 = local read "Cursor Windows by Trace"() -> (w1043:cluster{"start":dbl, "end":dbl}[])
        n509 = Index Array(array=w1043, index=w1044) -> (element=w1036:cluster{"start":dbl, "end":dbl})
        n510 = call <userlib>:"Offset 2D Trace.vi"("New Baseline"=w1042, "Ref Wind (ms)"=w1036, "Traces In"=w1041) -> ("Offset Traces Out"=w1039:cluster{"T0":sgl, "Delta T":sgl, "Data":sgl[][]})  [unwired: 1 in, 7 out]
        n511 = call <userlib>:"Offset 2D Trace.vi"("New Baseline"=w1042, "Ref Wind (ms)"=w1036, "Traces In"=w1040) -> ("Offset Traces Out"=w1038:cluster{"T0":sgl, "Delta T":sgl, "Data":sgl[][]})  [unwired: 1 in, 7 out]
        n512 = for {
          tunnel: w1031 -> [w1053]
          shift-right: [w1051] -> w1034
          shift-left: w1035 -> [w1052]
          tunnel: T20 {"Task"=enum."None", "Argument"=0} ("User Interface Tasks") -> [w1050]
          tunnel: w1033 -> [w1049] mode=indexing
          n513 = Bundle By Name(cluster=w1050, "Task"=w1049) -> (w1048:T20)
          n514 = Generate User Event(user event=w1053, event data cluster=w1048, error in=w1052) -> (error out=w1051:errorcluster)  [unwired: 1 in, 1 out]
        }
      }
      event "rectify": Mouse Down {
        n515 = event-data() -> ()  [unwired: 9 out]
        n516 = Unbundle By Name(w1063) -> ("Individual Data Sweeps"=w1066:sgl[][])
        n517 = Unbundle By Name(w1062) -> ("Individual Data Sweeps"=w1067:sgl[][])
        n518 = Generate User Event(user event=w1059, event data cluster=T20 {"Task"=enum."Plot Traces", "Argument"=0} ("User Interface Tasks")) -> ()  [unwired: 2 in, 2 out]
        n519 = Absolute Value(x=w1066) -> (abs(x)=w1065:sgl[][])
        n520 = Absolute Value(x=w1067) -> (abs(x)=w1064:sgl[][])
        n521 = Bundle By Name(cluster=w1063, "Individual Data Sweeps"=w1065) -> (w1061:T19)
        n522 = Bundle By Name(cluster=w1062, "Individual Data Sweeps"=w1064) -> (w1060:T19)
      }
      event "Avg Pts": Mouse Down {
        n523 = event-data() -> ()  [unwired: 9 out]
        n524 = call-poly <vilib>:"Mean.vi"("X"="Pts Around Yellow cursor") -> ("mean"=→"Pts Avg":dbl)  [unwired: 1 out]
      }
      event "cursors": Mouse Down {
        w1083 = sgl 0.0
        n525 = event-data() -> ()  [unwired: 9 out]
        n526 = property on="Graph 2" class="WFGraph (strict)"() -> ("Old Cursor List"=w1080:T34)  [unwired: 2 in, 2 out]
        n527 = case shown="\"2 filter\", Default" "cursor func" {
          tunnel: [w1093 w1098 w1104 w1111] -> w1085
          tunnel: [w1092 w1097 w1103 w1110] -> w1084
          tunnel: w1080 -> [_ w1102 w1108 w1113]
          frame "2 filter", Default {
            n528 = local read "Trace Processing Params"() -> (w1094:T6)
            n529 = Unbundle By Name(w1094) -> ("Filter Low Cut-off (Hz)"=w1093:dbl, "Filter High Cut-off (Hz)"=w1092:dbl)
            n530 = local write "Func Type"(enum16{"avg", "sum", "norm"}."norm" ("Func Type")) -> ()
          }
          frame "+- 10%" {
            n531 = call "graphCursor_info.vi"("Cursor List"=w1102) -> ("x0"=w1100:dbl)  [unwired: 1 in, 9 out]
            n532 = local write "Func Type"(enum16{"avg", "sum", "norm"}."sum" ("Func Type")) -> ()
            n533 = Multiply(x=w1100, y=sgl 0.1) -> (x*y=w1099:dbl)
            n534 = Add(x=w1100, y=w1099) -> (x+y=w1097:dbl)
            n535 = Subtract(x=w1100, y=w1099) -> (x-y=w1098:dbl)
          }
          frame "+- 5%" {
            n536 = call "graphCursor_info.vi"("Cursor List"=w1108) -> ("x0"=w1106:dbl)  [unwired: 1 in, 9 out]
            n537 = Multiply(x=w1106, y=sgl 0.05) -> (x*y=w1105:dbl)
            n538 = Add(x=w1106, y=w1105) -> (x+y=w1103:dbl)
            n539 = Subtract(x=w1106, y=w1105) -> (x-y=w1104:dbl)
          }
          frame "+-2" {
            w1109 = sgl -2.0 ("y")
            n540 = call "graphCursor_info.vi"("Cursor List"=w1113) -> ("x0"=w1112:dbl)  [unwired: 1 in, 9 out]
            n541 = Add(x=w1112, y=w1109) -> (x+y=w1110:dbl)
            n542 = Subtract(x=w1112, y=w1109) -> (x-y=w1111:dbl)
          }
        }
        n543 = Bundle("Filter Low Cut-off (Hz)"=w1085, w1083, "Filter High Cut-off (Hz)"=w1084, w1083) -> (w1082:T47)  [unwired: 1 out]
        n544 = call <userlib>:"2D to 1D Trace.vi"("2D Trace In"=w1079) -> ("1D Trace Out"=w1086:T37)  [unwired: 1 in, 3 out]
        n545 = call "Assign Cursor Coordinates.vi"("Trace1"=w1086, "Cursor Coordinate Assignments"=w1082, "Cursor List In"=w1080) -> ("Cursor List Out"=w1087:T48)  [unwired: 3 in, 5 out]
        n546 = property on="Graph 2" class="WFGraph (strict)"("Old Cursor List"=w1087) -> ()  [unwired: 2 in, 2 out]
      }
      event "Window Func": Mouse Down {
        n547 = event-data() -> ()  [unwired: 9 out]
        n548 = flat-sequence {
          tunnel: [w1126] -> w1115
          tunnel: [w1129] -> w1121
          tunnel: [w1128] -> w1116
          tunnel: w1115 -> [w1128]
          tunnel: w1121 -> [w1140]
          tunnel: w1120 -> [w1135]
          tunnel: [w1136] -> w1119
          tunnel: w1116 -> [w1134]
          frame #0 {
            n549 = property on="Graph 2" class="WFGraph (strict)"() -> ("Old Cursor List"=w1127:T34)  [unwired: 2 in, 2 out]
            n550 = call "graphCursor_info.vi"("Cursor List"=w1127) -> ("X pos"=w1126:cluster{"x0":dbl, "x1":dbl})  [unwired: 1 in, 9 out]
          }
          frame #1 {
            n551 = local read "Plot Flags 2"() -> (w1130:bool[])
            n552 = while {
              tunnel: w1130 -> [w1132] mode=indexing
              tunnel: [w1133] -> w1129
              i -> [w1133]
              stop <- w1131 continue-if-true
              n553 = Not(x=w1132) -> (.not. x?=w1131:bool)
            }
          }
          frame #2 {
            n554 = call <userlib>:"2D to 1D Trace.vi"("index"=w1140, "2D Trace In"=w1135) -> ("1D Trace Out"=w1139:T37)  [unwired: 3 out]
            n555 = call <userlib>:"Trace Subset-general.vi"("x0 zero?"=FALSE, "Wind (ms)"=w1134, "Trace"=w1139) -> ("Trace Out"=w1138:cluster{"x0":dbl, "dx":dbl, "Data":dbl[]})  [unwired: 1 in]
            n556 = case shown="\"sum\"" "Func Type" {
              tunnel: [w1144 w1150 0.0 ("mean")] -> w1142
              tunnel: w1138 -> [w1146 w1149 w1155]
              tunnel: [w1143 w1147 w1151] -> w1136
              tunnel: w1135 -> [w1143 w1147 _]
              frame "avg", Default {
                n557 = Unbundle By Name(w1146) -> ("Data"=w1145:dbl[])
                n558 = call-poly <vilib>:"Mean.vi"("X"=w1145) -> ("mean"=w1144:dbl)  [unwired: 1 out]
              }
              frame "sum" {
                n559 = Unbundle By Name(w1149) -> ("Data"=w1148:dbl[])
                n560 = Add Array Elements(numeric array=w1148) -> (sum=w1150:dbl)
              }
              frame "norm" {
                n561 = call <userlib>:"Normalize Trace.vi"("mode"=T25."sample norm", "Trace In"=w1155) -> ("Normalized Trace"=w1153:cluster{"T0":sgl, "Delta T":sgl, "Data":sgl[]})  [unwired: 4 in, 5 out]
                n562 = local write "cursor func"(enum16{"2 filter", "+- 10%", "+- 5%", "+-2"}."+- 10%" ("cursor func")) -> ()
                n563 = call <userlib>:"1D to 2D Trace.vi"("Trace In"=w1153) -> ("Trace Out"=w1151:cluster{"T0":sgl, "dT":sgl, "Data":sgl[][]})
              }
            }
            "Window Avg" <- w1142
          }
        }
        n564 = Generate User Event(user event=w1117, event data cluster=T20 {"Task"=enum."Plot Graph2", "Argument"=0} ("User Interface Tasks")) -> ()  [unwired: 2 in, 2 out]
      }
      event "Get Red Cursonr Pts": Mouse Down {
        n565 = event-data() -> ()  [unwired: 9 out]
        n566 = flat-sequence {
          tunnel: w1158 -> [w1164]
          frame #0 {
            n567 = property on="Graph 2" class="WFGraph (strict)"("Active Cursor"=u32 0) -> ()  [unwired: 2 in, 2 out]
          }
          frame #1 {
            n568 = Unbundle(w1164) -> ("T0"=w1166:sgl, "dT"=w1165:sgl, "Data"=w1174:sgl[][])
            n569 = property on="Graph 2" class="WFGraph (strict)"() -> ("Cursor.Cursor Position:Cursor X"=w1172:dbl)  [unwired: 2 in, 2 out]
            n570 = Index Array(array=w1174, index (row)=0) -> (element=w1168:sgl[])  [unwired: 1 in]
            n571 = call <userlib>:"x-units to index - trace.vi"("dx"=w1165, "x0"=w1166, "x"=w1172) -> ("Index"=w1170:i32)  [unwired: 2 in, 5 out]
            n572 = Decrement(x=w1170) -> (x-1=w1169:i32)
            n573 = Array Subset(array=w1168, index=w1169, length=3) -> (w1167:sgl[])
            n574 = local write "Pts Around Yellow cursor"(w1167) -> ()
          }
        }
      }
      event "Make window wrt Yel Cursor": Mouse Down {
        n575 = event-data() -> ()  [unwired: 9 out]
        n576 = local read "Graph 2 - cursor 0 x"() -> (w1177:sgl)
        n577 = stacked-sequence {
          tunnel: w1177 -> [_ _ w1184 _ _ w1190]
          frame #0 {
            n578 = property on="Graph 2" class="WFGraph (strict)"("Active Cursor"=u32 0) -> ()  [unwired: 2 in, 2 out]
          }
          frame #1 {
            n579 = property on="Graph 2" class="WFGraph (strict)"("Cursor.Cursor Lock Style"=u32 0 ("Cursor Locked")) -> ()  [unwired: 2 in, 2 out]
          }
          frame #2 {
            n580 = Multiply(x="Lower Factor", y=w1184) -> (x*y=w1185:sgl)
            n581 = property on="Graph 2" class="WFGraph (strict)"("Cursor.Cursor Position:Cursor X"=w1185) -> ()  [unwired: 2 in, 2 out]
          }
          frame #3 {
            n582 = property on="Graph 2" class="WFGraph (strict)"("Active Cursor"=u32 1) -> ()  [unwired: 2 in, 2 out]
          }
          frame #4 {
            n583 = property on="Graph 2" class="WFGraph (strict)"("Cursor.Cursor Lock Style"=u32 0 ("Cursor Locked")) -> ()  [unwired: 2 in, 2 out]
          }
          frame #5 {
            n584 = Multiply(x="Upper Factor", y=w1190) -> (x*y=w1189:sgl)
            n585 = property on="Graph 2" class="WFGraph (strict)"("Cursor.Cursor Position:Cursor X"=w1189) -> ()  [unwired: 2 in, 2 out]
          }
        }
      }
      event "cut traces": Mouse Down {
        n586 = event-data() -> ()  [unwired: 9 out]
        n587 = stacked-sequence {
          tunnel: w1200 -> [w1208 _]
          tunnel: w1199 -> [w1206 _]
          tunnel: [w1207 _] -> w1198
          tunnel: [w1205 _] -> w1197
          tunnel: w1196 -> [_ w1216]
          frame #0 {
            n588 = local read "Focus Mode"() -> (w1212:bool)
            n589 = case shown="True" w1212 {
              tunnel: [0 ("Focus") w1215] -> w1211
              frame False {
              }
              frame True {
                n590 = local read "Focus"() -> (w1215:i32)
                n591 = Decrement(x=w1215) -> (x-1=w1214:i32)
                n592 = local write "Old Focus"(w1214) -> ()
              }
            }
            n593 = local read "Cursor Windows by Trace"() -> (w1210:cluster{"start":dbl, "end":dbl}[])
            n594 = Index Array(array=w1210, index=w1211) -> (element=w1209:cluster{"start":dbl, "end":dbl})
            n595 = Unbundle By Name(w1209) -> ("start"=w1204:dbl, "end"=w1203:dbl)
            n596 = call <userlib>:"Trace Subset_2DTrace_v2.vi"("cut mode"="cut mode", "End"=w1203, "Start"=w1204, "Traces In"=w1208) -> ("Traces Out"=w1207:cluster{"T0":sgl, "Delta T":sgl, "Data":sgl[][]})  [unwired: 3 in]
            n597 = call <userlib>:"Trace Subset_2DTrace_v2.vi"("cut mode"="cut mode", "End"=w1203, "Start"=w1204, "Traces In"=w1206) -> ("Traces Out"=w1205:cluster{"T0":sgl, "Delta T":sgl, "Data":sgl[][]})  [unwired: 3 in]
          }
          frame #1 {
            # "If graph is not \"locked to point\", something happens with \"cursor windows by trace\" - it never is reassigned the new coordinates - it has something to do with frame 2 in lower left corner - if the case statement in that frame is never entered, then this works fine."
            # "alsways used cursor set 0!!!!"
            n598 = local read "Cursor Windows by Trace"() -> (w1223:cluster{"start":dbl, "end":dbl}[])
            n599 = property on="Trace A" class="WFGraph (strict)"() -> ("X Scale.Range"=w1220:T49)  [unwired: 2 in, 2 out]
            n600 = Unbundle By Name(w1220) -> ("Minimum"=w1219:dbl, "Maximum"=w1218:dbl)
            n601 = property on="Trace A" class="WFGraph (strict)"() -> ("Old Cursor List"=w1226:T34)  [unwired: 2 in, 2 out]
            n602 = Bundle("Minimum"=w1219, "Maximum"=w1218) -> (w1217:cluster{"Minimum":dbl, "Maximum":dbl})  [unwired: 1 out]
            n603 = Replace Array Subset "Replace Array Subset"(array=w1223, new element=w1217, index=0 ("Index")) -> (w1221:cluster{"start":dbl, "end":dbl}[])
            n604 = call <userlib>:"2D to 1D Trace.vi"("2D Trace In"=w1216) -> ("1D Trace Out"=w1225:T37)  [unwired: 1 in, 3 out]
            n605 = call "Assign Cursor Coordinates.vi"("Trace1"=w1225, "Mode"=T26."Default - Within Graph Range", "X Scale.Range"=w1220, "Cursor List In"=w1226) -> ("Cursor List Out"=w1224:T48)  [unwired: 2 in, 5 out]
            n606 = local write "Cursor Windows by Trace"(w1221) -> ()
            n607 = property on="Trace A" class="WFGraph (strict)"("Old Cursor List"=w1224) -> ()  [unwired: 2 in, 2 out]
          }
        }
        n608 = Generate User Event(user event=w1195, event data cluster=T20 {"Task"=enum."Plot Traces", "Argument"=0} ("User Interface Tasks")) -> ()  [unwired: 2 in, 2 out]
      }
      event "Shift by -500 except last traces": Mouse Down {
        n609 = event-data() -> ()  [unwired: 9 out]
        n610 = local read "Trace Ch Reference"() -> (w1234:enum16{"0", "1", "2", "3"})
        n611 = case shown="\"1\"" w1234 {
          tunnel: w1231 -> [w1260 _]
          tunnel: w1230 -> [_ w1261]
          tunnel: [w1260 w1261] -> w1235
          frame "0", Default {
          }
          frame "1" {
          }
        }
        n612 = Unbundle By Name(w1235) -> ("delta T"=w1239:sgl, "Individual Data Sweeps"=w1247:sgl[][])
        n613 = Array Size(array=w1247) -> (size(s)=w1250:i32[])
        n614 = Index Array(array=w1250, index=0) -> (element=w1248:i32)
        n615 = Subtract(x=w1248, y="Last #") -> (x-y=w1245:i32)
        n616 = Divide(x=500.0, y=w1239) -> (x/y=w1238:dbl)
        n617 = Delete From Array "Delete From Array"(array=w1247, length="Last #", index (row)=w1245) -> (deleted portion=w1243:sgl[][], array with subset deleted=w1244:sgl[][])  [unwired: 1 in]
        n618 = Generate User Event(user event=w1253, event data cluster=T20 {"Task"=enum."Plot Traces", "Argument"=0} ("User Interface Tasks"), error in=w1237) -> (error out=w1236:errorcluster)  [unwired: 1 in, 1 out]
        n619 = for {
          tunnel: w1244 -> [w1264] mode=indexing
          tunnel: [w1263] -> w1241 mode=indexing
          tunnel: w1238 -> [w1262]
          n620 = Delete From Array "Delete From Array"(array=w1264, length=w1262, index=0 ("disabled index (col)")) -> (array with subset deleted=w1263:sgl[])  [unwired: 1 out]
        }
        n621 = Build Array (concatenate)(w1241, w1243) -> (w1242:sgl[][])
        n622 = Bundle By Name(cluster=w1235, "Individual Data Sweeps"=w1242) -> (w1233:T19)
        n623 = case shown="\"1\"" w1234 {
          tunnel: w1233 -> [w1257 w1258]
          tunnel: [w1257 w1259] -> w1232
          tunnel: w1231 -> [_ w1259]
          tunnel: w1230 -> [w1256 _]
          tunnel: [w1256 w1258] -> w1229
          frame "0", Default {
          }
          frame "1" {
          }
        }
      }
      event "Set to A X-Axis", "Set to B X-Axis": Value Change {
        n624 = event-data() -> ()  [unwired: 7 out]
        n625 = case shown="True" "Set to A X-Axis" {
          frame False {
          }
          frame True {
            n626 = property on="Trace A" class="WFGraph (strict)"() -> ("X Scale.Old Range"=w1275:T50)  [unwired: 2 in, 2 out]
            n627 = property on="Graph 2" class="WFGraph (strict)"() -> ("X Scale.Old Range"=w1274:T50)  [unwired: 2 in, 2 out]
            n628 = property on="Time Course 2" class="IntGraph (strict)"("X Scale.Old Range"=w1274) -> ()  [unwired: 2 in, 2 out]
            n629 = property on="Time Course 1" class="IntGraph (strict)"("X Scale.Old Range"=w1274) -> ()  [unwired: 2 in, 2 out]
            n630 = property on="Trace B" class="WFGraph (strict)"("X Scale.Old Range"=w1275) -> ()  [unwired: 2 in, 2 out]
          }
        }
        n631 = case shown="True" "Set to B X-Axis" {
          frame False {
          }
          frame True {
            n632 = property on="Trace B" class="WFGraph (strict)"() -> ("X Scale.Old Range"=w1276:T50)  [unwired: 2 in, 2 out]
            n633 = property on="Trace A" class="WFGraph (strict)"("X Scale.Old Range"=w1276) -> ()  [unwired: 2 in, 2 out]
          }
        }
      }
      event "Trace A": Cursor Move; "Copy cursor window": Value Change {
        n634 = event-data() -> ()  [unwired: 5 out]
        n635 = stacked-sequence {
          seq-local: [_ w1296 _ _ _] -> [_ _ _ w1299 _]
          tunnel: [_ _ _ _ w1309] -> w1281
          frame #0 {
            w1295 = u32 0 ("Active Cursor")
            n636 = property on="Trace A" class="WFGraph (strict)"("Active Cursor"=w1295) -> ()  [unwired: 2 in, 2 out]
            n637 = property on="Trace B" class="WFGraph (strict)"("Active Cursor"=w1295) -> ()  [unwired: 2 in, 2 out]
          }
          frame #1 {
            n638 = property on="Trace A" class="WFGraph (strict)"() -> ("Cursor.Cursor Position:Cursor X"=w1296:dbl)  [unwired: 2 in, 2 out]
            n639 = property on="Trace B" class="WFGraph (strict)"("Cursor.Cursor Position:Cursor X"=w1296) -> ()  [unwired: 2 in, 2 out]
          }
          frame #2 {
            w1297 = u32 1 ("Active Cursor")
            n640 = property on="Trace B" class="WFGraph (strict)"("Active Cursor"=w1297) -> ()  [unwired: 2 in, 2 out]
            n641 = property on="Trace A" class="WFGraph (strict)"("Active Cursor"=w1297) -> ()  [unwired: 2 in, 2 out]
          }
          frame #3 {
            n642 = local read "Fix Wind Size"() -> (w1300:bool)
            n643 = case shown="False" w1300 {
              tunnel: [w1301 w1302] -> w1298
              tunnel: w1299 -> [_ w1303]
              frame False {
                n644 = property on="Trace A" class="WFGraph (strict)"() -> ("Cursor.Cursor Position:Cursor X"=w1301:dbl)  [unwired: 2 in, 2 out]
              }
              frame True {
                n645 = local read "Fixed Window Size"() -> (w1304:sgl)
                n646 = Add(x=w1303, y=w1304) -> (x+y=w1302:dbl)
              }
            }
            n647 = property on="Trace B" class="WFGraph (strict)"("Cursor.Cursor Position:Cursor X"=w1298) -> ()  [unwired: 2 in, 2 out]
            n648 = property on="Trace A" class="WFGraph (strict)"("Cursor.Cursor Position:Cursor X"=w1298) -> ()  [unwired: 2 in, 2 out]
          }
          frame #4 {
            n649 = property on="Trace B" class="WFGraph (strict)"() -> ("CrsrList"=w1306:T35)  [unwired: 2 in, 2 out]
            n650 = property on="Trace A" class="WFGraph (strict)"() -> ("CrsrList"=w1312:T35)  [unwired: 2 in, 2 out]
            n651 = call "graphCursor_info.vi"("Cursor List New Format"=w1312) -> ("dy"=→"dy A":sgl, "dx"=→"Window Size":sgl, "x1"=w1310:dbl, "x0"=w1311:dbl)  [unwired: 1 in, 6 out]
            n652 = call "graphCursor_info.vi"("Cursor List New Format"=w1306) -> ("dy"=→"dy B":sgl)  [unwired: 1 in, 9 out]
            n653 = Bundle("x0"=w1311, "x1"=w1310) -> (w1309:cluster{"x0":dbl, "x1":dbl})  [unwired: 1 out]
          }
        }
        n654 = Generate User Event(user event=w1278, event data cluster=T20 {"Task"=enum."Variable Update", "Argument"=0} ("User Interface Tasks")) -> ()  [unwired: 2 in, 2 out]
        n655 = case shown="True" "Copy cursor window" {
          tunnel: w1281 -> [_ w1287]
          frame False {
          }
          frame True {
            n656 = local read "Focus Mode"() -> (w1292:bool)
            n657 = case shown="True" w1292 {
              tunnel: [0 w1294] -> w1291
              frame False {
              }
              frame True {
                n658 = local read "Focus"() -> (w1294:i32)
              }
            }
            n659 = local read "Cursor Windows by Trace"() -> (w1289:cluster{"start":dbl, "end":dbl}[])
            n660 = local write "Message"("assign currsors" ("Message")) -> ()
            n661 = Replace Array Subset "Replace Array Subset"(array=w1289, new element=w1287, index=w1291) -> (w1288:cluster{"start":dbl, "end":dbl}[])
            n662 = local write "Cursor Windows by Trace"(w1288) -> ()
          }
        }
      }
      event "Graph 2": Cursor Move {
        n663 = event-data() -> ()  [unwired: 10 out]
        n664 = Generate User Event(user event=w1316, event data cluster=T20 {"Task"=enum."Variable Update", "Argument"=0} ("User Interface Tasks")) -> ()  [unwired: 2 in, 2 out]
      }
      event "Do Stats": Mouse Down {
        n665 = event-data() -> ()  [unwired: 9 out]
        n666 = local read "Stat Plot"() -> (w1342:cluster{dbl[], dbl[]}[])
        n667 = Index Array "Index Array"(array="Pair", index #1=0 ("index"), index #2=1 ("index")) -> (element #1=w1341:i32, element #2=w1340:i32)
        n668 = Index Array(array=w1342, index #1=w1341, index #2=w1340) -> (element #1=w1337:cluster{dbl[], dbl[]}, element #2=w1338:cluster{dbl[], dbl[]})
        n669 = Unbundle(w1337) -> (w1334:dbl[])  [unwired: 1 out]
        n670 = Unbundle(w1338) -> (w1326:dbl[])  [unwired: 1 out]
        n671 = case shown="True" "5 SD mark" {
          tunnel: w1326 -> [_ w1355]
          tunnel: [T28 {"+- factor*SD[0]"=-1000.0, "+- factor*SD[1]"=-1000.0} ("+- factor*SD") w1353] -> w1325
          frame False {
          }
          frame True {
            n672 = call "Normal Distrib. Stats.vi"("factor for SD"=5.0, "Samples"=w1355) -> ("+- factor*SD"=w1354:dbl[])  [unwired: 4 in, 5 out]
            n673 = Array To Cluster(array=w1354) -> (cluster=w1353:T28)
          }
        }
        n674 = call "2 sample Stat Comps.vi"("Sample 1"=w1326, "Sample 0"=w1334) -> ("Stat Results_Median"=→"Median Stats":T4, "Stat Results_Mean"=→"Stat Results_Mean":T3)  [unwired: 3 in, 5 out]
        n675 = case shown="\"Mean SE\"" "Mode" {
          tunnel: w1334 -> [_ w1368]
          tunnel: w1326 -> [_ w1367]
          tunnel: w1338 -> [w1356 _]
          tunnel: w1337 -> [w1357 _]
          tunnel: [w1358 w1359] -> w1336
          frame "Indiv", Default {
            n676 = Build Array(w1357, w1356) -> (w1358:cluster{dbl[], dbl[]}[])
          }
          frame "Mean SE" {
            w1366 = 0.0
            n677 = call "Normal Distrib. Stats.vi"("Samples"=w1368) -> ("mean +- Error"=w1365:dbl[])  [unwired: 5 in, 5 out]
            n678 = call "Normal Distrib. Stats.vi"("Samples"=w1367) -> ("mean +- Error"=w1362:dbl[])  [unwired: 5 in, 5 out]
            n679 = Build Array(w1366, w1366, w1366) -> (w1364:dbl[])
            n680 = Increment(x=w1364) -> (x+1=w1363:dbl[])
            n681 = Bundle(w1364, "mean +- Error"=w1365) -> (w1361:cluster{dbl[], "mean +- Error":dbl[]})  [unwired: 1 in]
            n682 = Bundle(w1363, "mean +- Error"=w1362) -> (w1360:cluster{dbl[], "mean +- Error":dbl[]})  [unwired: 1 in]
            n683 = Build Array(w1361, w1360) -> (w1359:cluster{dbl[], "mean +- Error":dbl[]}[])
          }
        }
        n684 = call-poly <vilib>:"Mean.vi"("X"=w1334) -> ("mean"=w1332:dbl)  [unwired: 1 out]
        n685 = call-poly <vilib>:"Mean.vi"("X"=w1326) -> ("mean"=w1333:dbl)  [unwired: 1 out]
        n686 = property on="Stat Plot" class="XYGraph (strict)"() -> ("CrsrList"=w1328:T35)  [unwired: 2 in, 2 out]
        n687 = Divide(x=w1333, y=w1332) -> (x/y=w1331:dbl)
        n688 = call "Assign Cursor Coordinates_LV8.vi"("Mode"=T27."Just Y coords", "Y Coords"=w1325, "Cursor List In"=w1328) -> ("Cursor List Out"=w1327:T35)  [unwired: 6 in, 2 out]
        n689 = Decrement(x=w1331) -> (x-1=w1330:dbl)
        n690 = property on="Stat Plot" class="XYGraph (strict)"("CrsrList"=w1327) -> ()  [unwired: 2 in, 2 out]
        n691 = local write "Stat Plot"(w1336) -> ()
        n692 = Build Array(w1332, w1333, w1330) -> (→"Means":dbl[])
      }
      event "Zoom": Mouse Down {
        n693 = event-data() -> ()  [unwired: 9 out]
        n694 = property on="Trace A" class="WFGraph (strict)"() -> ("Old Cursor List"=w1373:T34)  [unwired: 2 in, 2 out]
        n695 = call "graphCursor_info.vi"("Cursor List"=w1373) -> ("x1"=w1371:dbl, "x0"=w1372:dbl)  [unwired: 1 in, 8 out]
        n696 = property on="Trace A" class="WFGraph (strict)"("X Scale.Range:Minimum"=w1372, "X Scale.Range:Maximum"=w1371) -> ()  [unwired: 2 in, 2 out]
        n697 = property on="Trace B" class="WFGraph (strict)"("X Scale.Range:Minimum"=w1372, "X Scale.Range:Maximum"=w1371) -> ()  [unwired: 2 in, 2 out]
      }
      event "^2 four wind": Mouse Down {
        n698 = event-data() -> ()  [unwired: 9 out]
        n699 = local read "Time Course Window"() -> (w1386:sgl)
        n700 = Unbundle By Name(w1380) -> ("Delta T"=w1385:sgl)
        n701 = Quotient & Remainder(x=w1386, y=w1385) -> (floor(x/y)=w1383:sgl)  [unwired: 1 out]
        n702 = Increment(x=w1383) -> (x+1=w1384:sgl)
        n703 = call <userlib>:"Power_2_nearest.vi"("Number In"=w1384) -> ("Number Out"=w1382:sgl)  [unwired: 1 in, 2 out]
        n704 = Decrement(x=w1382) -> (x-1=w1381:sgl)
        n705 = Multiply(x=w1381, y=w1385) -> (x*y=w1387:sgl)
        n706 = local write "Time Course Window"(w1387) -> ()
      }
      event "Operate": Mouse Down {
        n707 = event-data() -> ()  [unwired: 9 out]
        n708 = Generate User Event(user event=w1392, event data cluster=T20 {"Task"=enum."Plot Graph2", "Argument"=0} ("User Interface Tasks")) -> ()  [unwired: 2 in, 2 out]
        n709 = local read "Trace Ch Reference"() -> (w1406:enum16{"0", "1", "2", "3"})
        n710 = call <userlib>:"2D Trace to TraceArray.vi"("2D Trace"=w1401) -> ("Trace Array"=w1409:cluster{"T0":sgl, "Delta T":sgl, "Data":sgl[]}[])
        n711 = call <userlib>:"2D Trace to TraceArray.vi"("2D Trace"=w1402) -> ("Trace Array"=w1398:cluster{"T0":sgl, "Delta T":sgl, "Data":sgl[]}[])
        n712 = Index Array(array=w1398, index="oper1") -> (element=w1396:cluster{"T0":sgl, "Delta T":sgl, "Data":sgl[]})
        n713 = Index Array(array=w1409, index="oper2") -> (element=w1407:cluster{"T0":sgl, "Delta T":sgl, "Data":sgl[]})
        n714 = Index Array(array=w1409, index="oper1") -> (element=w1408:cluster{"T0":sgl, "Delta T":sgl, "Data":sgl[]})
        n715 = Index Array(array=w1398, index="oper2") -> (element=w1397:cluster{"T0":sgl, "Delta T":sgl, "Data":sgl[]})
        n716 = call <userlib>:"Math Operate_Traces.vi"("operation"="operation", "Trace 2"=w1397, "Trace 1"=w1396) -> ("Trace Out"=w1404:cluster{"T0":sgl, "Delta T":sgl, "Data":sgl[]})  [unwired: 1 in, 7 out]
        n717 = call <userlib>:"Math Operate_Traces.vi"("operation"="operation", "Trace 2"=w1407, "Trace 1"=w1408) -> ("Trace Out"=w1405:cluster{"T0":sgl, "Delta T":sgl, "Data":sgl[]})  [unwired: 1 in, 7 out]
        n718 = case shown="\"1\"" w1406 {
          tunnel: w1405 -> [_ w1417]
          tunnel: w1404 -> [w1416 _]
          tunnel: [w1416 w1417] -> w1403
          frame "0", Default {
          }
          frame "1" {
          }
        }
        n719 = call <userlib>:"1D to 2D Trace.vi"("Trace In"=w1403) -> ("Trace Out"=w1394:cluster{"T0":sgl, "dT":sgl, "Data":sgl[][]})
        n720 = Build Array(w1396, w1397, w1404) -> (w1395:cluster{"T0":sgl, "Delta T":sgl, "Data":sgl[]}[])
        n721 = Build Array(w1408, w1407, w1405) -> (w1410:cluster{"T0":sgl, "Delta T":sgl, "Data":sgl[]}[])
        n722 = call <userlib>:"TraceArray to 2D Trace.vi"("Trace Array"=w1410) -> ("2D Trace"=w1399:cluster{"X0":sgl, "Delta X":sgl, "Data":sgl[][]})
        n723 = call <userlib>:"TraceArray to 2D Trace.vi"("Trace Array"=w1395) -> ("2D Trace"=w1400:cluster{"X0":sgl, "Delta X":sgl, "Data":sgl[][]})
      }
      event "AP Time Course": Mouse Down {
        n724 = event-data() -> ()  [unwired: 9 out]
        n725 = local read "Spikes Times A"() -> (w1421:T12)
        n726 = local read "Spike Times B"() -> (w1420:T12)
        n727 = case shown="\"cor\"" "AP Mode" {
          tunnel: w1421 -> [w1439 w1447 w1456]
          tunnel: w1420 -> [w1438 w1446 w1455]
          frame "cor" {
            n728 = local read "Window Size (ms)"() -> (w1436:sgl)
            n729 = local read "Trace Ch Reference"() -> (w1437:enum16{"0", "1", "2", "3"})
            n730 = local read "Normalization"() -> (w1434:enum16{"None", "Variance", "Sample Num"})
            n731 = global read "PowerCorrelation_globals.vi" "AP correl info"() -> (w1427:T39)
            n732 = local read "Corr Func"() -> (w1435:enum16{"Auto", "Cross"})
            n733 = local read "Time Course Increment"() -> (w1431:i32)
            n734 = local read "Time Course Window"() -> (w1432:sgl)
            n735 = Bundle("Corr Func"=w1435, "Window Size (ms)"=w1436, "Normalization"=w1434) -> (w1433:T41)  [unwired: 1 out]
            n736 = call "Avg Time Course Correlation.vi"("Spikes Times A"=w1439, "Spike Times B"=w1438, "Trace Focus"=w1437, "AP correl info"=w1427, "Time Course Increment (ms)"=w1431, "Moving Win Size (ms)"=w1432, "Correlation Parameters"=w1433) -> ("Time Course Data"=w1430:sgl[][], "x axis info out"=w1429:cluster{"x0":dbl, "dx":dbl}, "y axis info out"=w1428:cluster{"y0":dbl, "dy":dbl})  [unwired: 1 in, 9 out]
            n737 = local write "Time Course 1"(w1430) -> ()
            n738 = property on="Time Course 1" class="IntGraph (strict)"("X Scale.Offset and Multiplier"=w1429) -> ()  [unwired: 2 in, 2 out]
            n739 = property on="Time Course 1" class="IntGraph (strict)"("Y Scale.Offset and Multiplier"=w1428) -> ()  [unwired: 2 in, 2 out]
          }
          frame "coh" {
            n740 = local read "Time Course Increment"() -> (w1445:i32)
            n741 = global read "PowerCorrelation_globals.vi" "AP correl info"() -> (w1441:T39)
            n742 = Unbundle By Name(w1441) -> ("baseline Norm"=w1440:enum16{"none", "subtract", "divide"})
            n743 = local read "Time Course Window"() -> (w1444:sgl)
            n744 = call "Avg Time Course Coherence_spikeTimes.vi"("Spikes Times A"=w1447, "Spike Times B"=w1446, "Time Course Increment (ms)"=w1445, "baseline Norm"=w1440, "Moving Win Size (ms)"=w1444) -> ("Coherence time course"=w1443:cluster{"T0":sgl, "Delta T":sgl, "Data":sgl[]})  [unwired: 2 in, 12 out]
            n745 = call <userlib>:"1D to 2D Trace.vi"("Trace In"=w1443) -> ("Trace Out"=w1442:cluster{"T0":sgl, "dT":sgl, "Data":sgl[][]})
            n746 = local write "Graph 2"(w1442) -> ()
          }
          frame "Int/AP" {
            n747 = local read "Trace Ch Reference"() -> (w1449:enum16{"0", "1", "2", "3"})
            n748 = call "interval_spike_correlation_high.vi"("Interval Bin Size"="Int Bin", "Max Interval (ms)"="Max Interval", "Spike Bin Size (frac)"="AP Fract", "Interval Trace"=w1449, "Spike Times B"=w1455, "Spikes Times A"=w1456) -> ("y axis info out"=w1450:cluster{"y0":dbl, "dy":dbl}, "x axis info out"=w1451:cluster{"x0":dbl, "dx":dbl}, "Time Course Data"=w1452:sgl[][])  [unwired: 3 out]
            n749 = local write "Time Course 1"(w1452) -> ()
            n750 = property on="Time Course 1" class="IntGraph (strict)"("X Scale.Offset and Multiplier"=w1451) -> ()  [unwired: 2 in, 2 out]
            n751 = property on="Time Course 1" class="IntGraph (strict)"("Y Scale.Offset and Multiplier"=w1450) -> ()  [unwired: 2 in, 2 out]
          }
        }
      }
      event "Init Wind": Mouse Down {
        w1463 = cluster{sgl[], sgl, sgl}[] []
        n752 = event-data() -> ()  [unwired: 9 out]
        n753 = local write "Spike Times B"(w1463) -> ()
        n754 = local write "Spikes Times A"(w1463) -> ()
      }
      event "Add trace": Mouse Down {
        n755 = event-data() -> ()  [unwired: 9 out]
        n756 = local read "Focus"() -> (w1471:i32)
        n757 = Greater Or Equal To 0?(x=w1471) -> (x >= 0?=w1470:bool)
        n758 = case shown="True" w1470 {
          tunnel: w1467 -> [_ w1473]
          tunnel: w1466 -> [_ w1472]
          frame False {
          }
          frame True {
            w1476 = sgl 0.0
            w1488 = TRUE ("T0 zero?")
            w1489 = 0
            n759 = local read "Cursor Windows by Trace"() -> (w1495:cluster{"start":dbl, "end":dbl}[])
            n760 = local read "Focus"() -> (w1496:i32)
            n761 = Array Subset(array=w1495, index=w1496, length=1) -> (w1492:cluster{"start":dbl, "end":dbl}[])
            n762 = call <userlib>:"2D Trace to TraceArray.vi"("2D Trace"=w1472) -> ("Trace Array"=w1493:cluster{"T0":sgl, "Delta T":sgl, "Data":sgl[]}[])
            n763 = call <userlib>:"2D Trace to TraceArray.vi"("2D Trace"=w1473) -> ("Trace Array"=w1494:cluster{"T0":sgl, "Delta T":sgl, "Data":sgl[]}[])
            n764 = call <userlib>:"Trace Subset - TraceArray.vi"("Window by Trace"=w1492, "T0 zero?"=w1488, "Trace Array In"=w1493) -> ("Trace Array Out"=w1490:cluster{"X0":sgl, "dX":sgl, "Data":sgl[]}[])  [unwired: 1 in, 7 out]
            n765 = call <userlib>:"Trace Subset - TraceArray.vi"("Window by Trace"=w1492, "T0 zero?"=w1488, "Trace Array In"=w1494) -> ("Trace Array Out"=w1491:cluster{"X0":sgl, "dX":sgl, "Data":sgl[]}[])  [unwired: 1 in, 7 out]
            n766 = global read "Display & Avg Globals.vi" "spike trig params"() -> (w1474:T38)
            n767 = Index Array(array=w1490, index=w1489) -> (element=w1480:cluster{"X0":sgl, "dX":sgl, "Data":sgl[]})
            n768 = Index Array(array=w1491, index=w1489) -> (element=w1478:cluster{"X0":sgl, "dX":sgl, "Data":sgl[]})
            n769 = call "Get Spike Times.vi"("spike trig params"=w1474, "Trace"=w1478) -> ("Spike Times"=w1482:sgl[])  [unwired: 2 in, 7 out]
            n770 = call "Get Spike Times.vi"("spike trig params"=w1474, "Trace"=w1480) -> ("Spike Times"=w1481:sgl[])  [unwired: 2 in, 7 out]
            n771 = call <userlib>:"Trace Length.vi"("Trace"=w1478) -> ("Length (x-units)"=w1477:sgl)  [unwired: 4 out]
            n772 = call <userlib>:"Trace Length.vi"("Trace"=w1480) -> ("Length (x-units)"=w1479:sgl)  [unwired: 4 out]
            n773 = Bundle("Spike Times"=w1481, w1476, "Length (x-units)"=w1479) -> (w1483:T51)  [unwired: 1 out]
            n774 = Bundle("Spike Times"=w1482, w1476, "Length (x-units)"=w1477) -> (w1485:T51)  [unwired: 1 out]
            n775 = Build Array (concatenate)("Spike Times B", w1483) -> (w1486:T52)
            n776 = Build Array (concatenate)("Spikes Times A", w1485) -> (w1487:T52)
            n777 = local write "Spike Times B"(w1486) -> ()
            n778 = local write "Spikes Times A"(w1487) -> ()
          }
        }
      }
      event "Cursor Near Spike": Mouse Down {
        n779 = event-data() -> ()  [unwired: 9 out]
        n780 = local read "Trace Ch Reference"() -> (w1528:enum16{"0", "1", "2", "3"})
        n781 = local read "Cursor Windows by Trace"() -> (w1527:cluster{"start":dbl, "end":dbl}[])
        n782 = case shown="\"0\", Default" w1528 {
          tunnel: [w1529 w1530] -> w1526
          tunnel: w1501 -> [w1529 _]
          tunnel: w1500 -> [_ w1530]
          frame "0", Default {
          }
          frame "1" {
          }
        }
        n783 = local read "Focus"() -> (w1507:i32)
        n784 = Array Subset(array=w1527, index=w1507, length=1) -> (w1524:cluster{"start":dbl, "end":dbl}[])
        n785 = call <userlib>:"2D Trace to TraceArray.vi"("2D Trace"=w1526) -> ("Trace Array"=w1525:cluster{"T0":sgl, "Delta T":sgl, "Data":sgl[]}[])
        n786 = call <userlib>:"Trace Subset - TraceArray.vi"("Window by Trace"=w1524, "T0 zero?"=FALSE, "Trace Array In"=w1525) -> ("Trace Array Out"=w1522:cluster{"X0":sgl, "dX":sgl, "Data":sgl[]}[])  [unwired: 1 in, 7 out]
        n787 = global read "Display & Avg Globals.vi" "spike trig params"() -> (w1504:T38)
        n788 = Index Array(array=w1522, index=0) -> (element=w1520:cluster{"X0":sgl, "dX":sgl, "Data":sgl[]})
        n789 = property on="Trace A" class="WFGraph (strict)"() -> ("Old Cursor List"=w1515:T34)  [unwired: 2 in, 2 out]
        n790 = call "Get Spike Times.vi"("spike trig params"=w1504, "Trace"=w1520) -> ("Spike Times"=w1519:sgl[])  [unwired: 2 in, 7 out]
        n791 = call "graphCursor_info.vi"("Cursor List"=w1515) -> ("y1"=w1509:dbl, "y0"=w1510:dbl, "x1"=w1512:dbl)  [unwired: 1 in, 7 out]
        n792 = Index Array(array=w1519, index=0) -> (element=w1517:sgl)
        n793 = Subtract(x=w1517, y=sgl 2.0) -> (x-y=w1511:sgl)
        n794 = Bundle(w1511, "y0"=w1510, "x1"=w1512, "y1"=w1509) -> (w1508:cluster{sgl, "y0":dbl, "x1":dbl, "y1":dbl})  [unwired: 1 out]
        n795 = call <userlib>:"2D to 1D Trace.vi"("2D Trace In"=w1502) -> ("1D Trace Out"=w1505:T37)  [unwired: 1 in, 3 out]
        n796 = call "Assign Cursor Coordinates.vi"("Trace1"=w1505, "Mode"=T26."Assign given coordinates", "Cursor Coordinate Assignments"=w1508, "Cursor List In"=w1515) -> ("Cursor List Out"=w1513:T48)  [unwired: 2 in, 5 out]
        n797 = property on="Trace A" class="WFGraph (strict)"("Old Cursor List"=w1513) -> ()  [unwired: 2 in, 2 out]
      }
      event "Shuffle Trace": Mouse Down {
        n798 = event-data() -> ()  [unwired: 9 out]
        n799 = call <userlib>:"2D to 1D Trace.vi"("2D Trace In"=w1535) -> ("1D Trace Out"=w1539:T37)  [unwired: 1 in, 3 out]
        n800 = call <userlib>:"Shuffle Trace.vi"("Shuffle Window Size (ms)"=sgl 2000.0, "Trace In"=w1539) -> ("Shuffled Trace"=w1537:cluster{"t0":sgl, "dT":sgl, "Data":sgl[]})  [unwired: 3 out]
        n801 = call <userlib>:"1D to 2D Trace.vi"("Trace In"=w1537) -> ("Trace Out"=w1534:cluster{"T0":sgl, "dT":sgl, "Data":sgl[][]})
      }
      event "Dump Cursor Wind", "Load Cursor Wind": Value Change {
        n802 = event-data() -> ()  [unwired: 7 out]
        n803 = local read "File Paths"() -> (w1541:T9)
        n804 = case shown="True" "Dump Cursor Wind" {
          tunnel: w1541 -> [_ w1565]
          frame False {
          }
          frame True {
            n805 = Unbundle By Name(w1565) -> ("Anal Path"=w1566:path)
            n806 = call "File Dialog"("start path"=w1566, "default name"="x.wCurs", "pattern (all files)"="*.wCurs" ("default name")) -> ("selected path"=w1564:path)  [unwired: 4 in, 8 out]
            n807 = local read "Cursor Windows by Trace"() -> (w1572:cluster{"start":dbl, "end":dbl}[])
            n808 = Open/Create/Replace Datalog(5:cluster{"start":sgl, "end":sgl}[] [] ("Cursor Windows by Trace"), 10:T29."replace or create" ("operation (0:open)"), 11:w1564) -> (0:w1576:errorcluster, 3:w1573:refnum<k1>)  [unwired: 1 in, 3 out]
            n809 = Write Datalog(4:w1576, 6:w1572, 7:w1573) -> (0:w1575:errorcluster, 3:w1570:refnum<k1>)
            n810 = Close File(refnum=w1570, error in=w1575) -> (error out=w1574:errorcluster)  [unwired: 1 out]
            n811 = call <vilib>:"General Error Handler.vi"("error in (no error)"=w1574) -> ()  [unwired: 2 in, 13 out]
            n812 = Bundle By Name(cluster=w1565, "Anal Path"=w1564) -> (w1563:T9)
            n813 = local write "File Paths"(w1563) -> ()
          }
        }
        n814 = case shown="True" "Load Cursor Wind" {
          tunnel: w1541 -> [_ w1552]
          frame False {
          }
          frame True {
            n815 = Unbundle By Name(w1552) -> ("Anal Path"=w1553:path)
            n816 = call "File Dialog2"("start path"=w1553, "pattern (all files)"="*.wCurs" ("default name")) -> ("selected path"=w1551:path)  [unwired: 5 in, 8 out]
            n817 = Open/Create/Replace Datalog(5:cluster{"start":sgl, "end":sgl}[] [] ("Cursor Windows by Trace"), 10:T29."open" ("operation (0:open)"), 11:w1551) -> (0:w1557:errorcluster, 3:w1562:refnum<k1>)  [unwired: 1 in, 3 out]
            n818 = Read Datalog(4:w1557, 7:w1562) -> (0:w1558:errorcluster, 2:w1556:cluster{"start":sgl, "end":sgl}[], 3:w1560:refnum<k1>)  [unwired: 1 out]
            n819 = local write "Cursor Windows by Trace"(w1556) -> ()
            n820 = Close File(refnum=w1560, error in=w1558) -> (error out=w1559:errorcluster)  [unwired: 1 out]
            n821 = call <vilib>:"General Error Handler.vi"("error in (no error)"=w1559) -> ()  [unwired: 2 in, 13 out]
            n822 = Bundle By Name(cluster=w1552, "Anal Path"=w1551) -> (w1550:T9)
            n823 = local write "Assign Cursors In Plot"(FALSE ("Assign Cursors Flag")) -> ()
            n824 = local write "File Paths"(w1550) -> ()
          }
        }
      }
      event "One Cursor Window": Mouse Down {
        n825 = event-data() -> ()  [unwired: 9 out]
        n826 = Generate User Event(user event=w1578, event data cluster=T20 {"Task"=enum."Variable Update", "Argument"=0} ("User Interface Tasks")) -> ()  [unwired: 2 in, 2 out]
      }
      event "Time Course 1": Cursor Move {
        n827 = event-data() -> ()  [unwired: 10 out]
        n828 = case shown="True" "Cursor Slave\nTime Course" {
          frame False {
          }
          frame True {
            n829 = property on="Time Course 2" class="IntGraph (strict)"() -> ("Old Cursor List"=w1593:T42)  [unwired: 2 in, 2 out]
            n830 = property on="Time Course 1" class="IntGraph (strict)"() -> ("Old Cursor List"=w1592:T42)  [unwired: 2 in, 2 out]
            n831 = call "Assign Cursor Coordinates_IntensGraph.vi"("Cursor List Target"=w1593, "Cursor List Source"=w1592) -> ("Cursor List Out"=w1594:T48)  [unwired: 5 out]
            n832 = property on="Time Course 2" class="IntGraph (strict)"("Old Cursor List"=w1594) -> ()  [unwired: 2 in, 2 out]
          }
        }
      }
      event "Up State Analysis": Mouse Down {
        n833 = event-data() -> ()  [unwired: 9 out]
        n834 = local read "File Paths"() -> (w1598:T9)
        n835 = local read "Trace Processing Params"() -> (w1596:T6)
        n836 = local read "File Info"() -> (w1603:T7)
        n837 = Build Array(w1602, w1601) -> (w1600:T2)
        n838 = local read "Strings"() -> (w1595:T1)
        n839 = call "upstate_wind_12.21.17.vi"("Strings"=w1595, "Trace Processing Params"=w1596, "File Paths In"=w1598, "File Info"=w1603, "Original Traces - all Chan"=w1599, "Processed Traces - all Chan"=w1600) -> ("File Paths Out"=w1597:T9)  [unwired: 3 in]
        n840 = local write "File Paths"(w1597) -> ()
      }
      event "Prog Info", "Correlation Params": Value Change {
        n841 = event-data() -> ()  [unwired: 7 out]
        n842 = case shown="True" "Correlation Params" {
          frame False {
          }
          frame True {
            n843 = call "Correlation Params Panel.vi"() -> ()  [unwired: 6 out]
          }
        }
        n844 = case shown="True" "Prog Info" {
          frame False {
          }
          frame True {
            n845 = call "Info-PowerSpec.vi"() -> ()  [unwired: 1 out]
          }
        }
      }
      event "Trace Export": Mouse Down {
        n846 = event-data() -> ()  [unwired: 9 out]
        n847 = global read "Analysis Globals.vi" "File Times"() -> (w1618:string[])
        n848 = local read "File Paths"() -> (w1623:T9)
        n849 = Index Array(array=w1618) -> (element=w1617:string)  [unwired: 1 in]
        n850 = case shown="\"Graph 2\"" "Export Graph" {
          tunnel: [w1631 w1640 w1659 w1670] -> w1619
          tunnel: w1623 -> [w1630 w1639 w1656 w1673]
          tunnel: "Export Name" -> [w1629 w1633 w1651 w1662]
          tunnel: w1622 -> [_ w1637 w1655 _]
          tunnel: w1621 -> [_ w1636 w1654 _]
          tunnel: w1617 -> [w1628 w1634 w1652 w1663]
          frame "Graph 2" {
            n851 = local read "Graph 2"() -> (w1632:cluster{"T0":sgl, "delta T":sgl, sgl[][]})
            n852 = local read "Analysis Notes"() -> (w1627:string)
            n853 = call "Trace Dump - Standard.vi"("Date:Time"=w1628, "Filename prefix"=w1629, "Hidden Notes"=w1627, "File Paths In"=w1630, "Trace"=w1632) -> ("File Paths Out"=w1631:T9)  [unwired: 2 in, 4 out]
          }
          frame "traces (focus)" {
            n854 = local read "Focus"() -> (w1642:i32)
            n855 = call <userlib>:"2D to 1D Trace.vi"("index"=w1642, "2D Trace In"=w1637) -> ("1D Trace Out"=w1644:T37)  [unwired: 3 out]
            n856 = call <userlib>:"2D to 1D Trace.vi"("index"=w1642, "2D Trace In"=w1636) -> ("1D Trace Out"=w1643:T37)  [unwired: 3 out]
            n857 = Build Array(w1644, w1643) -> (w1641:T53)
            n858 = case shown="True" FALSE {
              tunnel: w1642 -> [_ w1650]
              tunnel: w1641 -> [w1645 w1648]
              tunnel: [w1645 w1647] -> w1638
              frame False {
              }
              frame True {
                n859 = local read "Cursor Windows by Trace"() -> (w1649:cluster{"start":dbl, "end":dbl}[])
                n860 = Index Array(array=w1649, index=w1650) -> (element=w1646:cluster{"start":dbl, "end":dbl})
                n861 = call <userlib>:"Trace Subset - TraceArray.vi"("Subset Wind (ms)"=w1646, "Trace Array In"=w1648) -> ("Trace Array Out"=w1647:cluster{"X0":sgl, "dX":sgl, "Data":sgl[]}[])  [unwired: 3 in, 6 out]
              }
            }
            n862 = call "Trace Dump - Standard.vi"("Date:Time"=w1634, "Filename prefix"=w1633, "File Paths In"=w1639, "Trace Array"=w1638) -> ("File Paths Out"=w1640:T9)  [unwired: 3 in, 4 out]
          }
          frame "All Traces (Ref)" {
            n863 = local read "Trace Ch Reference"() -> (w1658:enum16{"0", "1", "2", "3"})
            n864 = case shown="\"0\", Default" w1658 {
              tunnel: [w1660 w1661] -> w1657
              tunnel: w1655 -> [w1660 _]
              tunnel: w1654 -> [_ w1661]
              frame "0", Default {
              }
              frame "1" {
              }
            }
            n865 = call <userlib>:"2D Trace to TraceArray.vi"("2D Trace"=w1657) -> ("Trace Array"=w1653:cluster{"T0":sgl, "Delta T":sgl, "Data":sgl[]}[])
            n866 = call "Trace Dump - Standard.vi"("Date:Time"=w1652, "Filename prefix"=w1651, "File Paths In"=w1656, "Trace Array"=w1653) -> ("File Paths Out"=w1659:T9)  [unwired: 3 in, 4 out]
          }
          frame "Color Graph 1" {
            w1675 = sgl 0.0
            n867 = property on="Time Course 1" class="IntGraph (strict)"() -> ("X Scale.Offset and Multiplier"=w1669:T43)  [unwired: 2 in, 2 out]
            n868 = property on="Time Course 1" class="IntGraph (strict)"() -> ("Y Scale.Offset and Multiplier"=w1666:T43)  [unwired: 2 in, 2 out]
            n869 = local read "Time Course 1"() -> (w1676:sgl[][])
            n870 = Unbundle By Name(w1666) -> ("Offset"=w1665:dbl, "Multiplier"=w1664:dbl)
            n871 = Unbundle By Name(w1669) -> ("Offset"=w1668:dbl, "Multiplier"=w1667:dbl)
            n872 = Bundle(w1675, w1675, "Time Course 1"=w1676) -> (w1674:cluster{sgl, sgl, "Time Course 1":sgl[][]})  [unwired: 1 out]
            n873 = Format Into String(format string="x0 %.2f, dx %.2f, y0 %.2f, dy %.2f", w1668, w1667, w1665, w1664) -> (resulting string=w1671:string)  [unwired: 2 in, 1 out]
            n874 = call "Trace Dump - Standard.vi"("Date:Time"=w1663, "Filename prefix"=w1662, "Hidden Notes"=w1671, "File Paths In"=w1673, "Trace"=w1674) -> ("File Paths Out"=w1670:T9)  [unwired: 2 in, 4 out]
          }
        }
        n875 = local write "File Paths"(w1619) -> ()
      }
      event "Quit": Mouse Down {
        n876 = event-data() -> ()  [unwired: 9 out]
        n877 = Not(x="Quit") -> (.not. x?=w1683:bool)
      }
    }
  }
  n878 = Destroy User Event(user event=w4, error in=w3) -> (error out=w7:errorcluster)
  n879 = Unregister For Events(event registration refnum=w2, error in=w7) -> (error out=w6:errorcluster)
  n880 = call <vilib>:"Simple Error Handler.vi"("error in (no error)"=w6) -> ()  [unwired: 4 in, 5 out]
